vi "TLB Native Dynamic Events ver 0.13c.vi"() -> ()   [LabVIEW 2018]
uses:
  Labview Training Phase 2/Enum Controls/States for Action Engine.ctl
  TLB Type Definitions/State Type Definitions, for 0.26d versions and later.ctl
  TLB Type Definitions/Intruction Type Definitions.ctl
  TLB Type Definitions/Encoder cluster.ctl
  TLB Type Definitions/PING CLUSTER.ctl
  <vilib>/Studica/Studica Toolkit/NavX/NavX.lvlib
  <vilib>/Studica/Studica Toolkit/Background/DIO Channel.ctl
  Underlying VI's/NavX VI/navX type def.ctl
  <vilib>/myRIO/Instrument Drivers/Utilities/Utilities.lvlib
  <vilib>/Studica/Studica Toolkit/Background/I2C Channel.ctl
  TLB Type Definitions/Vision cluster.ctl
  <vilib>/NI_Real-Time Target Support.lvlib
  TLB Type Definitions/Stepper cluster.ctl
  Experimental VI's/Archived VI's/MOTOR CONTROL NO PID Type Def.ctl
  Underlying VI's/I2C Master VI/I2C MASTER Type Def.ctl
  Underlying VI's/I2C Master VI/I2C_MASTER_WRITE_NEW Type Def.ctl
  Underlying VI's/Webcam FGV Low level ver/State control.ctl
  <vilib>/userdefined/High Color/IMAQdx.ctl
  Underlying VI's/I2C Master VI/Arduino_Interfacing.ctl
  <vilib>/Studica/Studica Toolkit/NavX/TypeDefs/Flags/Z900_navX_Flags_CalibrationStatusTypeDef.ctl
  <vilib>/Studica/Studica Toolkit/NavX/TypeDefs/Flags/Z900_navX_Flags_OpStatusTypeDef.ctl
  <vilib>/Utility/RT CPU Load.ctl
panel:
  out "Arduino Data":T1
  out "CPU loads":T2[](array[typedef]) {"ISR (%)" format="%#.2f"; "Idle (%)" format="%#.2f"; "Background (%)" format="%#.2f"; "Normal (%)" format="%#.2f"; "Above Normal (%)" format="%#.2f"; "High (%)" format="%#.2g"; "Timed Structures (%)" format="%#.2g"; "Time Critical (%)" format="%#.2g"; "Total (%)" format="%#.2g"}
  in  "Red LED":bool
  out "Object Center Coordinates":cluster{"x":sgl, "y":sgl}
  out "Object detection cluster":T3
  in  "Mode":enum16{"Ball", "Soap", "Gel", "Pipe", "None"}(ring)
  out "Detect?":bool
  out "Status":T6 {"OP Status" items=["INITIALIZING", "SELFTEST_IN_PROGRESS", "ERROR", "IMU_AUTOCAL_IN_PROGRESS", "NORMAL"]; "Calibration Status" items=["IMU_CAL_STATE_MASK"=3, "IMU_CAL_STATE_INPROGRESS"=0, "IMU_CAL_STATE_ACCUMULATE"=1, "IMU_CAL_STATE_COMPLETE"=2]}
  out "NavX Readings":T7
  out "TASK ENABLE":bool
  out "Rising Edge":bool
  in  "Green LED":bool
  out "Object detected?":bool
  out "I2C Error":errorcluster
  out "Speed & distance":T8
  out "State Logic":T9=enum."Startup"
  out "elements":T10[](array[typedef])
  in  "STOP TASK":bool
  in  "OK Button":bool
  in  "STOP":bool
  out "error out":errorcluster
  out "Action Queue Items":i32
  out "State Logic Queue Items":i32
  out "Action Queues items":string[](array[string])=["Hardware reset", "Software reset", ""]
  out "Action State":string
  # "TLB FRAMEWORK STATUS"
  # "System Health Status Update"
  # "Test Programme written by Calvin Loke    Dated: 28 Aug 2019\nTest Programme revised by Dr Alex See   Dated 30 Aug 2019\n\nProgramme version:   TLB Native Dynamic Events ver 0.04b.vi"
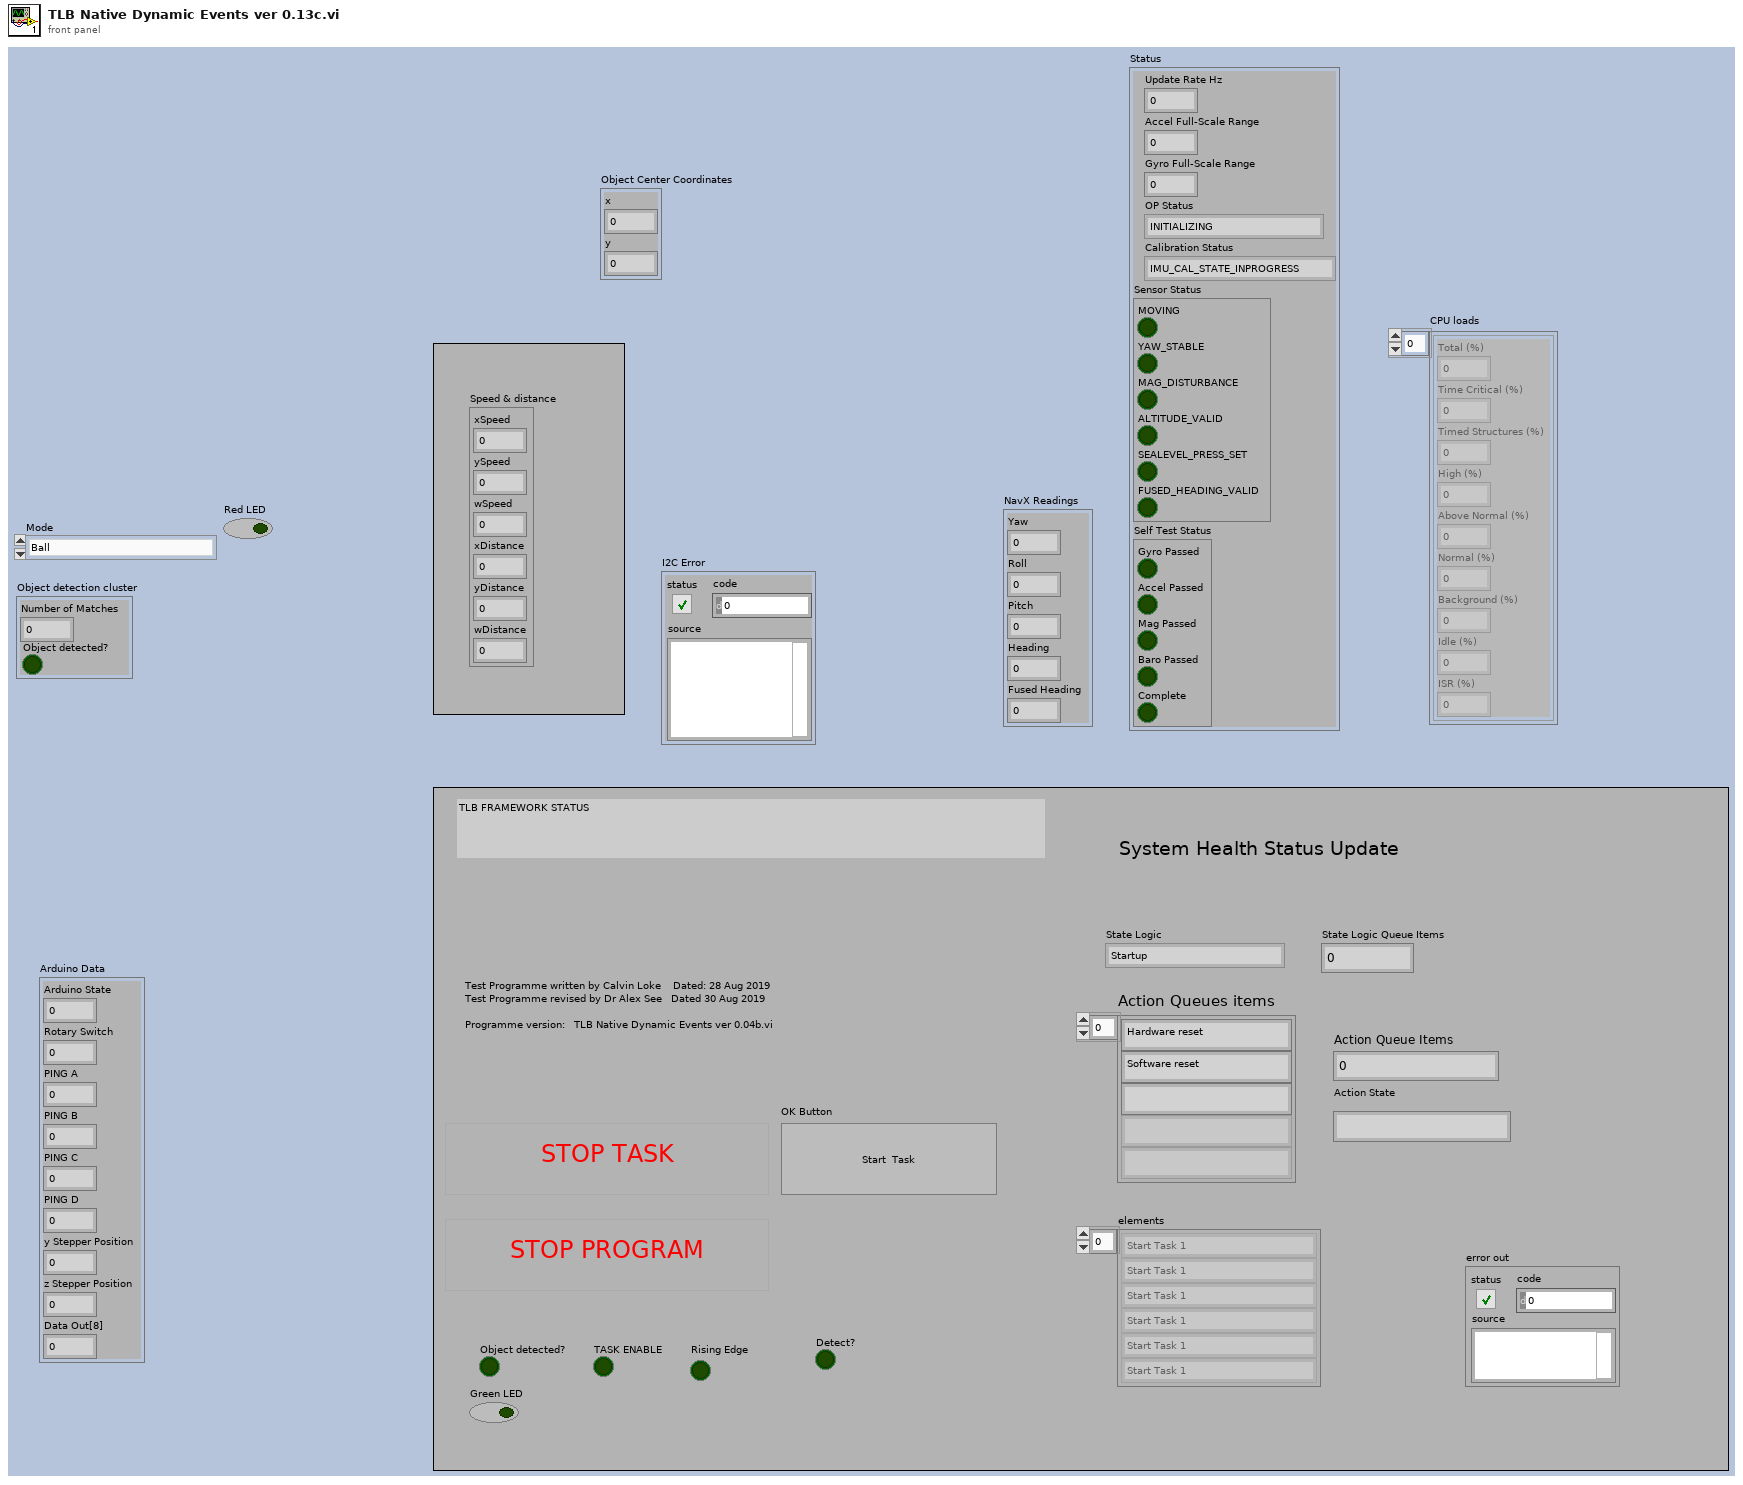
[diagram p1: front panel]
types:
  T1 = cluster{"Arduino State":u8, "Rotary Switch":u8, "PING A":u8, "PING B":u8, "PING C":u8, "PING D":u8, "y Stepper Position":u8, "z Stepper Position":u8, "Data Out[8]":u8}
  T2 = typedef "NI_Real-Time Target Support.lvlib/RT CPU Load.ctl" = cluster{"Total (%)":dbl, "Time Critical (%)":dbl, "Timed Structures (%)":dbl, "High (%)":dbl, "Above Normal (%)":dbl, "Normal (%)":dbl, "Background (%)":dbl, "Idle (%)":dbl, "ISR (%)":dbl}
  T3 = cluster{"Number of Matches":i32, "Object detected?":bool}
  T4 = typedef "NavX.lvlib/Z900_navX_Flags_OpStatusTypeDef.ctl" = u8
  T5 = typedef "NavX.lvlib/Z900_navX_Flags_CalibrationStatusTypeDef.ctl" = u8
  T6 = cluster{"Update Rate Hz":u8, "Accel Full-Scale Range":u8, "Gyro Full-Scale Range":u16, "OP Status":T4, "Calibration Status":T5, "Sensor Status":cluster{"MOVING":bool, "YAW_STABLE":bool, "MAG_DISTURBANCE":bool, "ALTITUDE_VALID":bool, "SEALEVEL_PRESS_SET":bool, "FUSED_HEADING_VALID":bool}, "Self Test Status":cluster{"Gyro Passed":bool, "Accel Passed":bool, "Mag Passed":bool, "Baro Passed":bool, "Complete":bool}}
  T7 = cluster{"Yaw":dbl, "Roll":dbl, "Pitch":dbl, "Heading":dbl, "Fused Heading":dbl}
  T8 = cluster{"xSpeed":dbl, "ySpeed":dbl, "wSpeed":dbl, "xDistance":dbl, "yDistance":dbl, "wDistance":dbl}
  T9 = typedef "State Type Definitions.ctl" = enum16{"None", "Startup", "Move to Angle", "True Stop", "Idle", "Shutdown", "Task 1A", "Task 1B", "Task 2:Raise Arm", "Task 2:Sensor Mode", "Task 2:Reverse Mode", "Task 3", "Task 4_A", "Task 4_B", "Task 4_C", "Task 4_D", "Task 5A", "Task 5B", "Task 5C", "Task 5D", "Task 5E: POSITION ARM", "Task 5F: ARM GRAB HEIGHT", "Task 5G: CLOSE CLAW", "Task 5H: RAISE ARM", "Task 6_A", "Task 6_B", "Task 7", "Task 8A: RAISE ARM", "Task 8B: MOVE TO BOX", "Task 8C: CAM BURST", "Task 8D: PROCESS IMAGE", "Task 8E: ROBOT ADJUST", "Task 8F: CAM BURST 2", "Task 8G: PROCESS IMAGE 2", "Task 8H: ARM ADJUST", "Task 8I: ARM GRAB HEIGHT", "Task 8J: CLOSE CLAW", "Task 8K: RAISE MY SWORD", "Task 9A: Raise Arm", "Task 9B: Rotate to Angle", "Task 9C: Detect Box", "Task 9D: MOVE FORWARD", "Task 9E: MOVE LEFT", "Task 9F: SCAN IMAGE", "Task 9G: PROCESS COLOUR", "Task 9H: MOVE RIGHT", "Task 9I: SCAN IMAGE", "Task 9J: PROCESS COLOUR", "Task 9K: ROTATE 90 CW", "Task 9L: MOVE FORWARD", "Task 9M: MOVE RIGHT", "Task 9N: SCAN IMAGE", "Task 9O: PROCESS COLOUR", "Task 9P: MOVE RIGHT", "Task 9Q: SCAN IMAGE", "Task 9R: PROCESS COLOUR", "Task A1: Raise Arm", "Task A2: Rotate to Angle", "Task A3: Move Forward", "Task A4: Rotate CW 90"}
  T10 = typedef "Intruction Type Definitions.ctl" = enum16{"None", "Start Task 1", "Start Task 2", "Start Task 3", "Start Task 4", "Start Task 5", "Start Task 6", "Start Task 7", "Start Task 8 - BALL", "Start Task 8 - Gel", "Start Task 8 - Pipe", "Start Task 8 - Soap", "Start Task 9", "Start Task A", "Start Task B", "Exit"}
  T11 = typedef "States for Action Engine.ctl" = enum16{"Initialize", "Write", "Read"}
  T12 = typedef "Stepper cluster.ctl" = cluster{"y Stepper Position":u8, "z Stepper Position":u8}
  T13 = typedef "DIO Channel.ctl" = enum16{"Not Connected", "A/DIO1", "A/DIO2", "A/DIO3", "A/DIO4", "A/DIO5", "A/DIO6", "A/DIO7", "A/DIO13", "B/DIO1", "B/DIO2", "B/DIO3", "B/DIO4", "B/DIO5", "B/DIO6", "B/DIO7", "B/DIO13", "C/DIO0", "C/DIO1", "C/DIO2", "C/DIO3", "C/DIO4", "C/DIO5", "C/DIO6", "C/DIO7"}
  T14 = typedef "Vision cluster.ctl" = cluster{"Recognized Object":bool, "Object X coordinate":dbl, "Object Y coordinate":dbl}
  T15 = typedef "PING CLUSTER.ctl" = cluster{"PING_A":u8, "PING_B":u8, "PING_C":u8, "PING_D":u8}
  T16 = typedef "Encoder cluster.ctl" = cluster{"xDistance":dbl, "yDistance":dbl, "wDistance":dbl}
  T17 = typedef "Arduino_Interfacing.ctl" = enum16{"Initialize", "Write to Arduino", "Read From Arduino"}
  T18 = typedef "I2C Channel.ctl" = enum16{"Not Connected", "A", "B"}
  T19 = typedef "navX type def.ctl" = enum16{"Get i2C reference", "Read Values", "Zero Yaw"}
  T20 = typedef "State Type Definitions.ctl" = enum16{"None", "Startup", "Move to Angle", "True Stop", "Idle", "Shutdown", "Task 1", "Task 2:Raise Arm", "Task 2:Sensor Mode", "Task 2:Reverse Mode", "Task 3", "Task 4_A", "Task 4_B", "Task 4_C", "Task 4_D", "Task 5A: ARM CAM HEIGHT", "Task 5B: MOVE TO BOX", "Task 5C: CAM BURST", "Task 5D: PROCESS IMAGE", "Task 5E: POSITION ARM", "Task 5F: ARM GRAB HEIGHT", "Task 5G: CLOSE CLAW", "Task 5H: RAISE ARM", "Task 6_A", "Task 6_B", "Task 7", "Task 8A: RAISE ARM", "Task 8B: MOVE TO BOX", "Task 8C: CAM BURST", "Task 8D: PROCESS IMAGE", "Task 8E: ROBOT ADJUST", "Task 8F: CAM BURST 2", "Task 8G: PROCESS IMAGE 2", "Task 8H: ARM ADJUST", "Task 8I: ARM GRAB HEIGHT", "Task 8J: CLOSE CLAW", "Task 8K: RAISE MY SWORD", "Task 9A: Raise Arm", "Task 9B: Rotate to Angle", "Task 9C: Detect Box", "Task 9D: MOVE FORWARD", "Task 9E: MOVE LEFT", "Task 9F: SCAN IMAGE", "Task 9G: PROCESS COLOUR", "Task 9H: MOVE RIGHT", "Task 9I: SCAN IMAGE", "Task 9J: PROCESS COLOUR", "Task 9K: ROTATE 90 CW", "Task 9L: MOVE FORWARD", "Task 9M: MOVE RIGHT", "Task 9N: SCAN IMAGE", "Task 9O: PROCESS COLOUR", "Task 9P: MOVE RIGHT", "Task 9Q: SCAN IMAGE", "Task 9R: PROCESS COLOUR"}
  T21 = typedef "State Type Definitions.ctl" = enum16{"None", "Startup", "Move to Angle", "True Stop", "Idle", "Shutdown", "Task 1", "Task 2", "Task 3", "Task 4_A", "Task 4_B", "Task 4_C", "Task 5", "Task 6_A", "Task 6_B", "Task 7", "Task 8", "Task 9", "Task A", "Task B"}
  T22 = typedef "MOTOR CONTROL NO PID Type Def.ctl" = enum16{"Init", "Front Back", "Left Right", "Rotate", "Stop", "Latch"}
  T23 = typedef "I2C_MASTER_WRITE_NEW Type Def.ctl" = enum16{"Ultrasonic sensors", "Stepper origin", "zStepper 13.3k", "zStepper 13k", "zStepper 12k", "zStepper 11k", "zStepper 10k", "zStepper 9k", "zStepper 8k", "zStepper 7k", "zStepper 6k", "zStepper 5k", "zStepper 4k", "zStepper 3k", "zStepper 2k", "zStepper 1k", "zStepper 900", "zStepper 800", "zStepper 700", "zStepper 600", "zStepper 500", "zStepper 400", "zStepper 300", "zStepper 200", "zStepper 100", "zStepper 0", "yStepper control", "Open Claw", "Close Claw", "Soft Reset"}
  T24 = typedef "State control.ctl" = enum16{"Initialise", "Start camera", "Continuous Acquisition ", "Stop camera", "Dispose all"}
  T25 = typedef "IMAQdx.ctl" = refnum<k21>
  T26 = cluster{"DIO Channel":T13, "FPGA VI Reference Out":refnum<k20>}
  T27 = cluster{"I2C Ref Out":cluster{"I2C Channel":T18, "FPGA VI Reference Out":refnum<k20>}, "Connected":bool, "Slave Address (7-bit)":u8, "Registry":u8[]}
  T28 = typedef "IMAQ Image.ctl" = refnum<image>
  T29 = typedef "I2C MASTER Type Def.ctl" = enum16{"Last State", "Mode 0", "Mode 1", "Mode 2", "Mode 3", "Mode 4", "Mode 5", "Mode 6", "Mode 7", "Mode 8", "Mode 9", "Mode 10"}
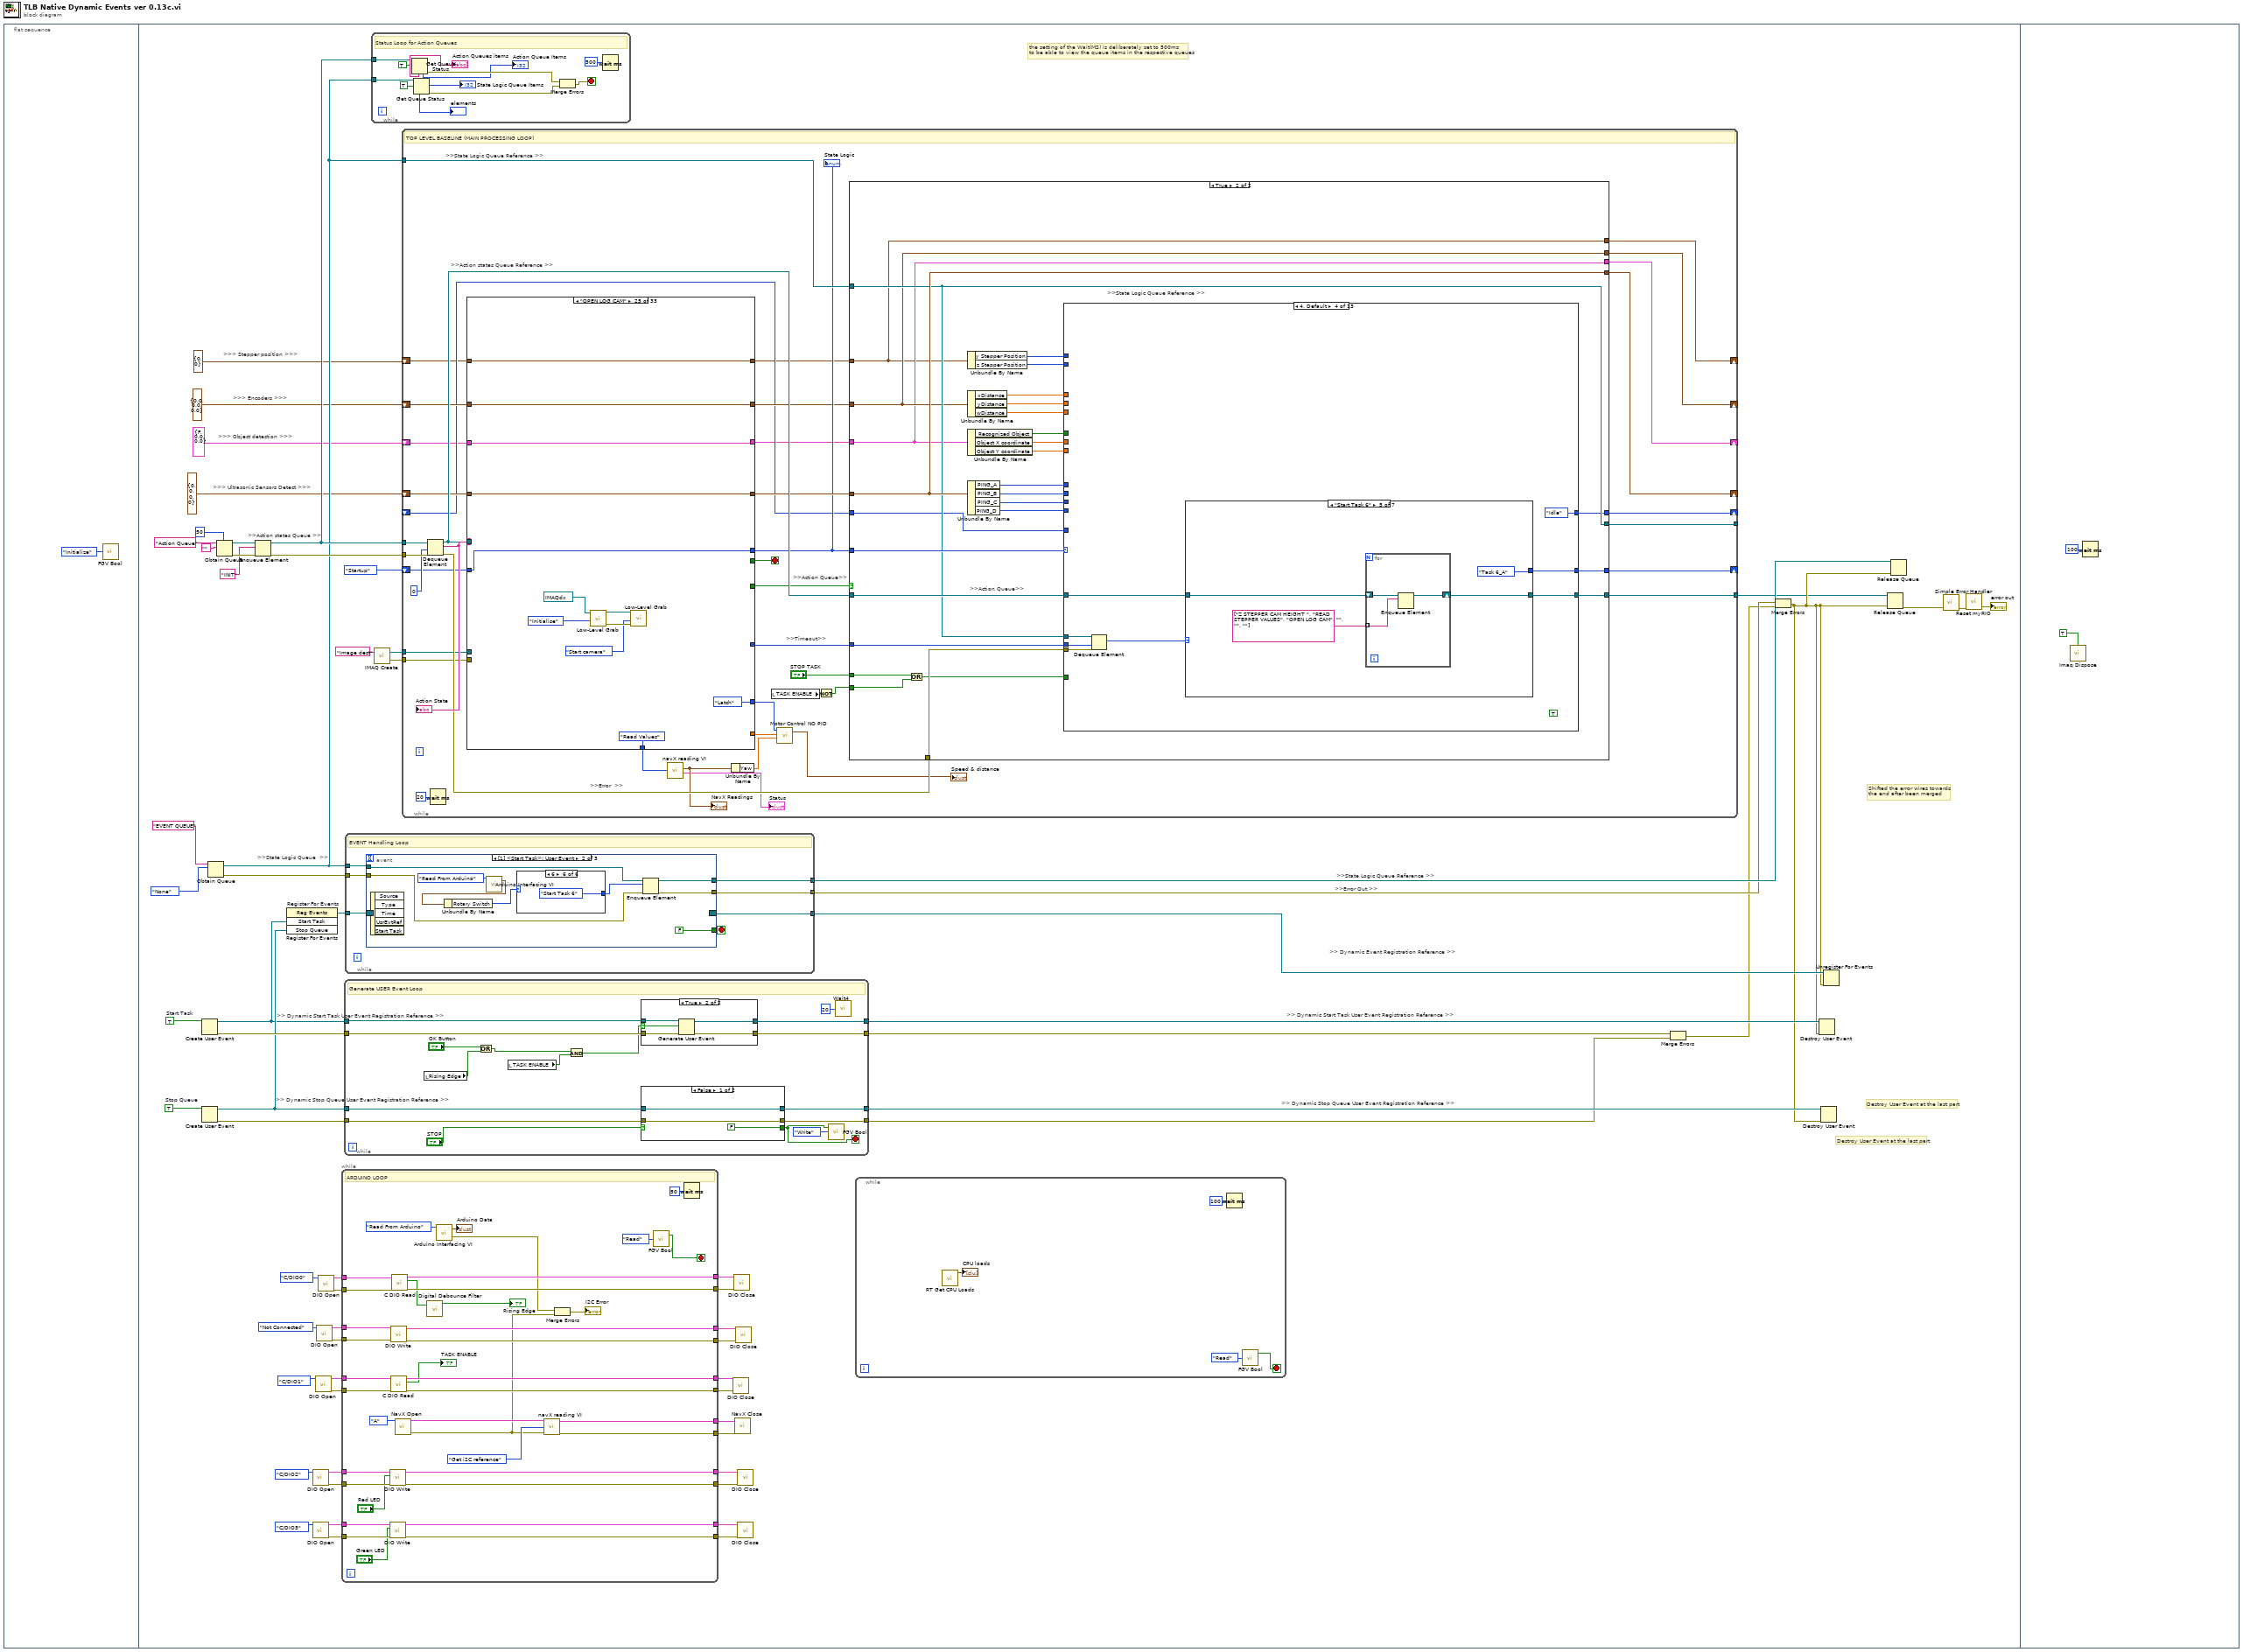
[diagram p0: block diagram]
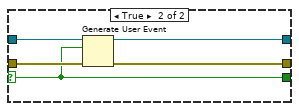
[diagram p2: hidden frame]
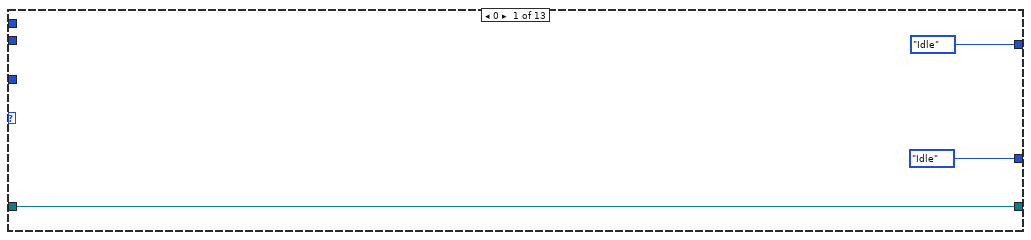
[diagram p5: hidden frame]
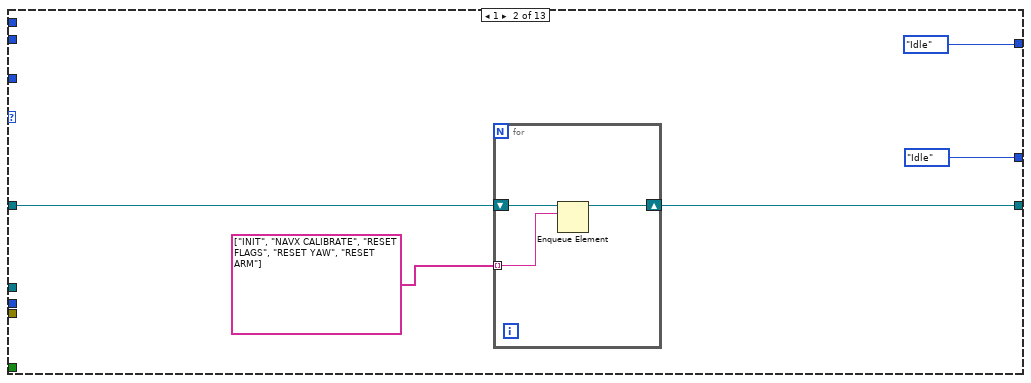
[diagram p6: hidden frame]
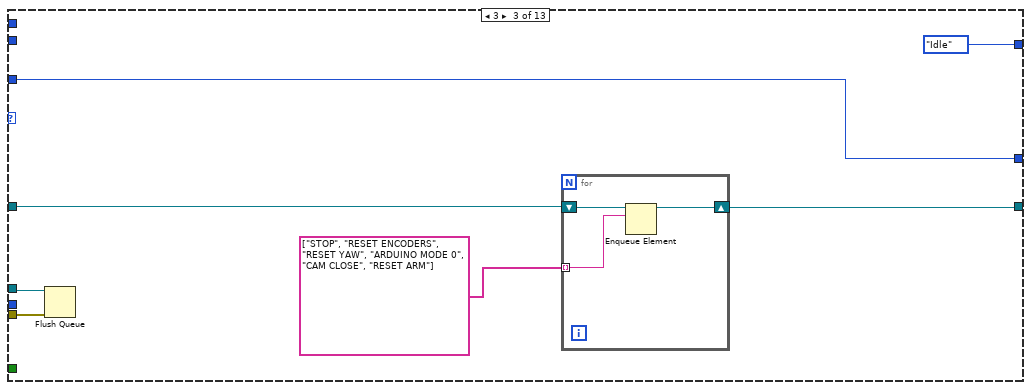
[diagram p7: hidden frame]
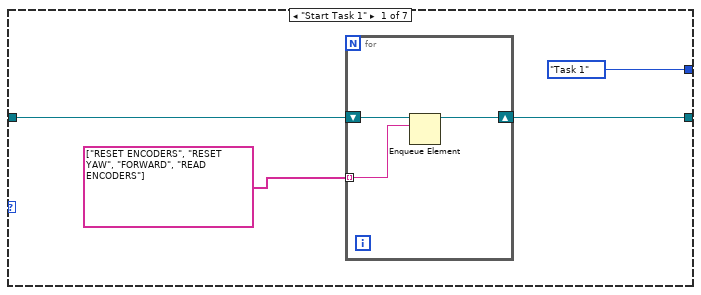
[diagram p8: hidden frame]
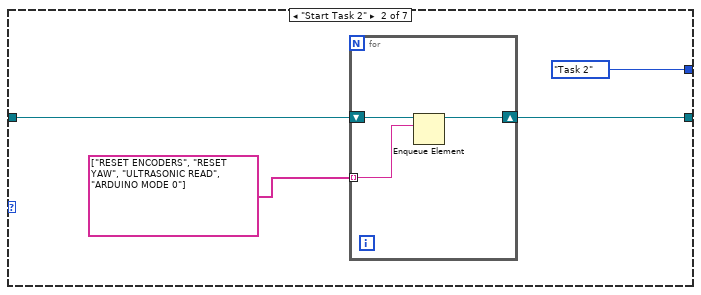
[diagram p9: hidden frame]
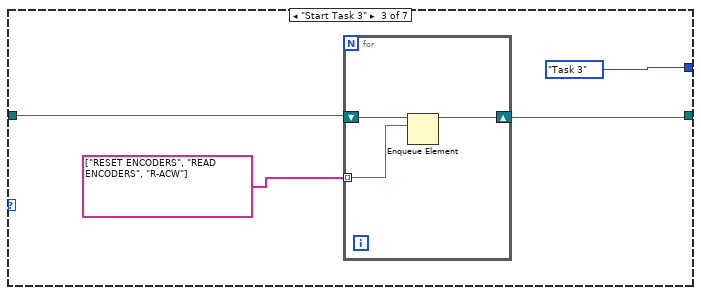
[diagram p10: hidden frame]
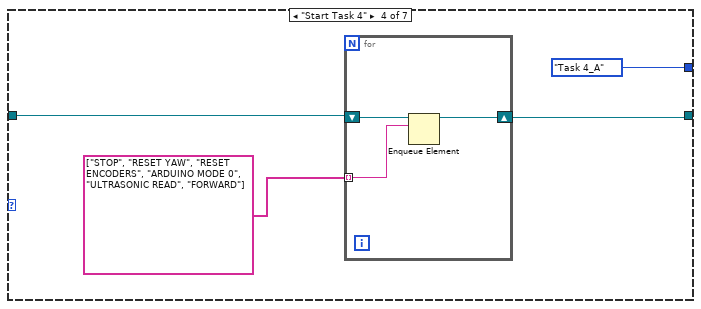
[diagram p11: hidden frame]
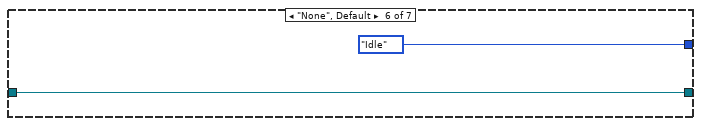
[diagram p12: hidden frame]
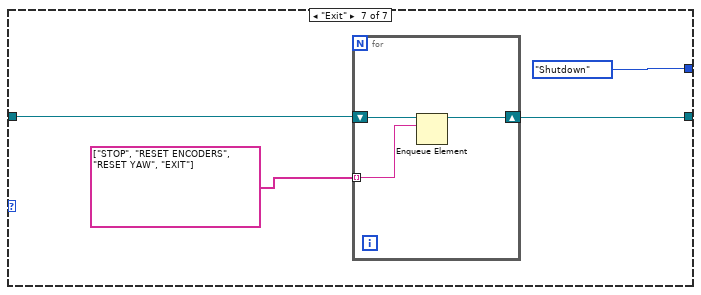
[diagram p13: hidden frame]
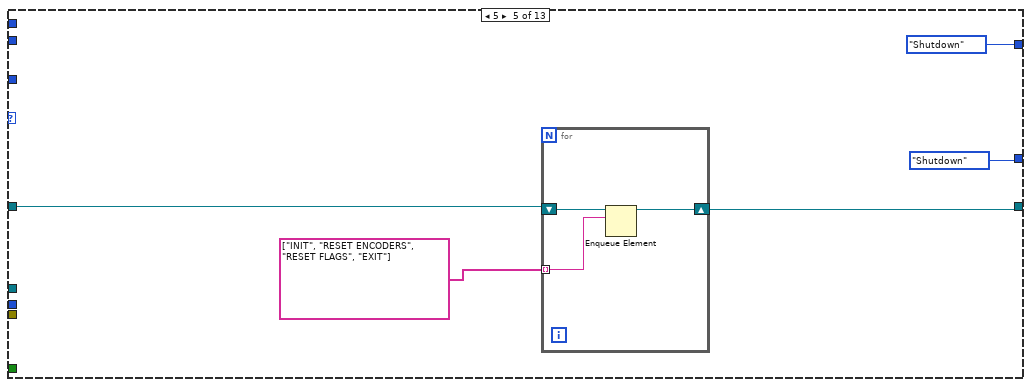
[diagram p14: hidden frame]
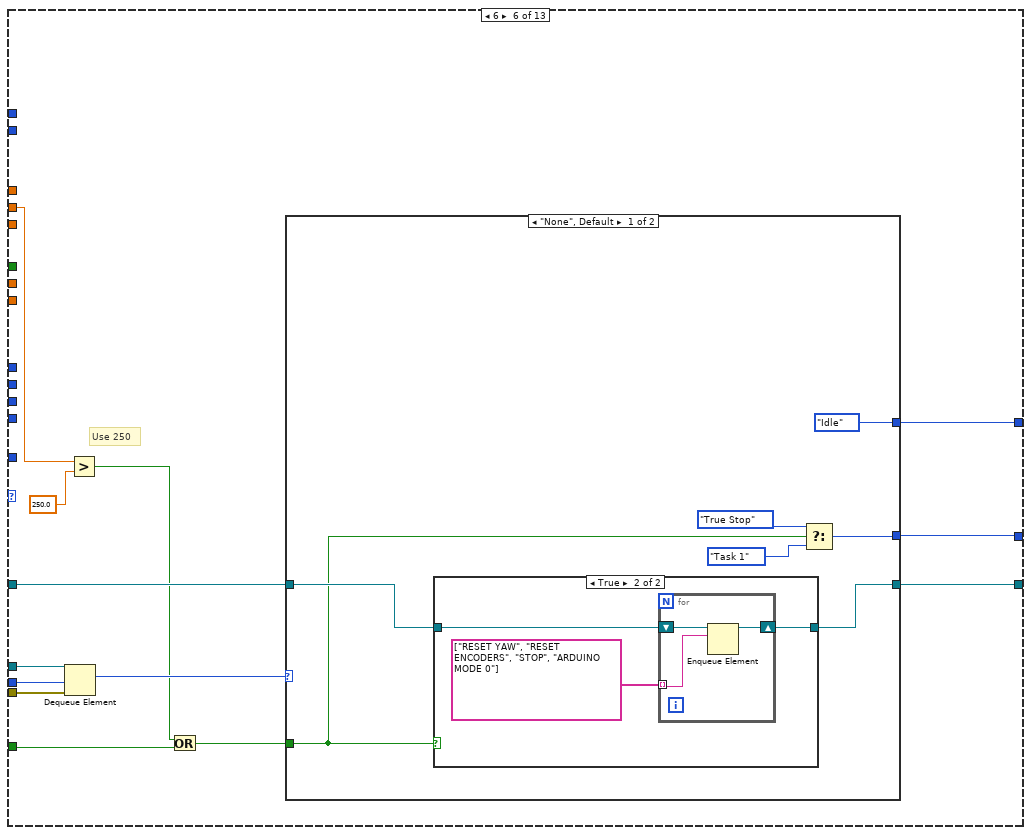
[diagram p15: hidden frame]
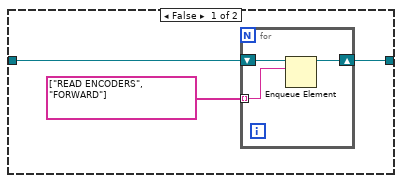
[diagram p16: hidden frame]
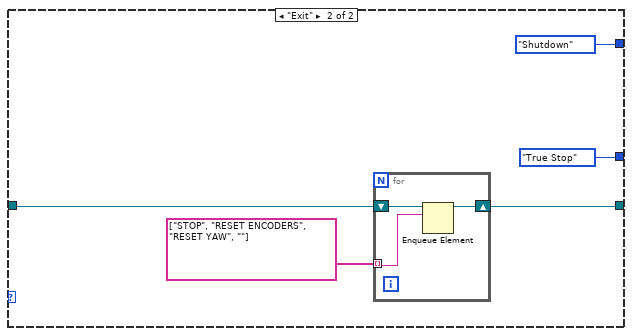
[diagram p17: hidden frame]
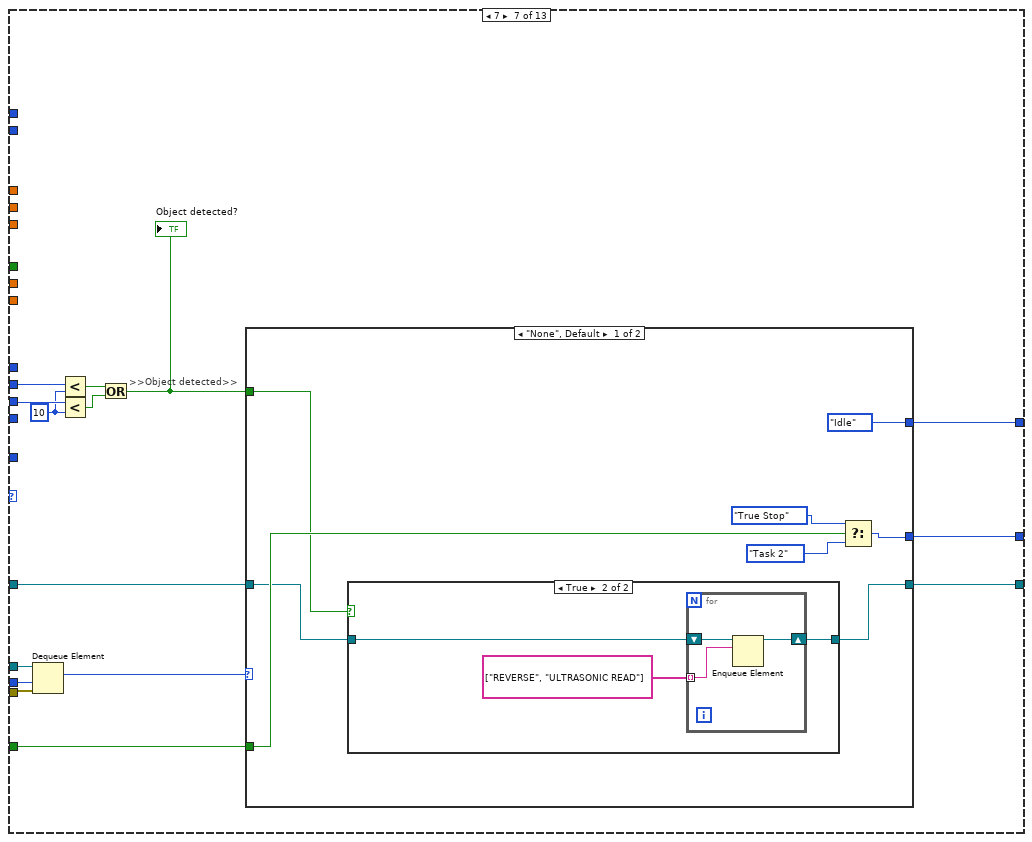
[diagram p18: hidden frame]
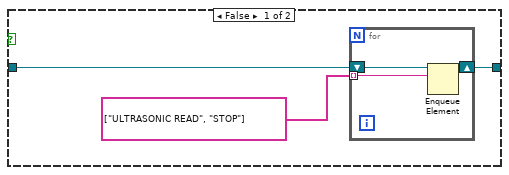
[diagram p19: hidden frame]
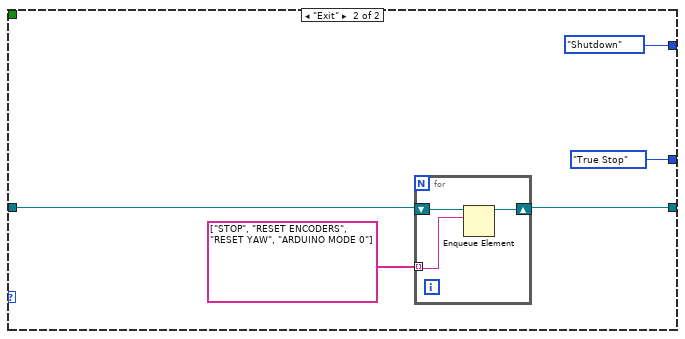
[diagram p20: hidden frame]
diagram:
  n1 = flat-sequence {
    frame #0 {
      n2 = call "FGV Bool.vi"("Init/Read/Write State"=States_for_Action_Engine."Initialize") -> ()  [unwired: 2 in, 2 out]
    }
    frame #1 {
      w68 = TRUE  # Stop Queue
      w67 = TRUE  # Start Task
      # ">>> Stepper position >>>"
      # ">>> Encoders >>>"
      # ">>> Object detection >>>"
      # ">>> Ultrasonic Sensors Detect >>>"
      # "the setting of the Wait(MS) is deliberately set to 500ms\nto be able to view the queue items in the respective queues"
      # ">>Error Out >>"
      # ">> Dynamic Stop Queue User Event Registration Reference >>"
      # ">> Dynamic Start Task User Event Registration Reference >>"
      # ">> Dynamic Stop Queue User Event Registration Reference >>"
      # ">> Dynamic Start Task User Event Registration Reference >>"
      # ">> Dynamic Event Registration Reference >>"
      # ">>Action states Queue >>"
      # ">>State Logic Queue  >>"
      # ">>State Logic Queue Reference >>"
      # "Destroy User Event at the last part"
      # "Destroy User Event at the last part"
      # "Shifted the error wires towards\nthe end after been merged"
      n3 = Create User Event(user event datatype=w67) -> (user event=w59:refnum<user-event>, error out=w64:errorcluster)  [unwired: 1 in]
      n4 = Create User Event(user event datatype=w68) -> (user event=w60:refnum<user-event>, error out=w63:errorcluster)  [unwired: 1 in]
      n5 = Obtain Queue(name (unnamed)="EVENT QUEUE", element data type=Intruction_Type_Definitions."None" ("Enum")) -> (queue out=w45:refnum<queue>, error out=w51:errorcluster)  [unwired: 3 in, 1 out]
      n6 = Obtain Queue(max queue size (-1, unlimited)=50, name (unnamed)="Action Queue", element data type="") -> (queue out=w54:refnum<queue>, error out=w50:errorcluster)  [unwired: 2 in, 1 out]
      n7 = Enqueue Element(queue=w54, element="INIT", error in (no error)=w50) -> (queue out=w46:refnum<queue>, error out=w49:errorcluster)  [unwired: 1 in, 1 out]
      n8 = register-events "Register For Events"(w59, w60) -> (reference out=w58:refnum<event-registration>)  [unwired: 2 in, 1 out]
      n9 = call <vilib>:"DIO Open.vi"("DIO Channel"=DIO_Channel."C/DIO2") -> ("error out"=w10:errorcluster, "DIO Info Out"=w11:T26)  [unwired: 9 in]
      n10 = call <vilib>:"DIO Open.vi"("DIO Channel"=DIO_Channel."C/DIO3") -> ("error out"=w5:errorcluster, "DIO Info Out"=w6:T26)  [unwired: 9 in]
      n11 = call <vilib>:"DIO Open.vi"("DIO Channel"=DIO_Channel."C/DIO1") -> ("error out"=w23:errorcluster, "DIO Info Out"=w24:T26)  [unwired: 9 in]
      n12 = call <vilib>:"DIO Open.vi"("DIO Channel"=DIO_Channel."Not Connected") -> ("error out"=w28:errorcluster, "DIO Info Out"=w30:T26)  [unwired: 9 in]
      n13 = call <vilib>:"DIO Open.vi"("DIO Channel"=DIO_Channel."C/DIO0") -> ("error out"=w33:errorcluster, "DIO Info Out"=w36:T26)  [unwired: 9 in]
      n14 = while {
        tunnel: w36 -> [w107]
        tunnel: [w106] -> w34
        tunnel: w33 -> [w105]
        tunnel: [w104] -> w32
        tunnel: w30 -> [w100]
        tunnel: [w99] -> w29
        tunnel: w28 -> [w98]
        tunnel: [w97] -> w27
        tunnel: [w96] -> w25
        tunnel: w24 -> [w95]
        tunnel: w23 -> [w94]
        tunnel: [w93] -> w22
        tunnel: [w90] -> w21
        tunnel: [w89] -> w20
        tunnel: w11 -> [w85]
        tunnel: w10 -> [w84]
        tunnel: [w83] -> w9
        tunnel: [w82] -> w8
        tunnel: w6 -> [w80]
        tunnel: w5 -> [w79]
        tunnel: [w78] -> w4
        tunnel: [w77] -> w3
        stop <- w109 stop-if-true
        # "ARDUINO LOOP"
        n15 = call <vilib>:"DIO Write.vi"("error in (no error)"=w84, "Input"="Red LED", "DIO Info In"=w85) -> ("error out"=w82:errorcluster, "DIO Info Out"=w83:T26)  [unwired: 7 in]
        n16 = call <vilib>:"DIO Write.vi"("error in (no error)"=w79, "Input"="Green LED", "DIO Info In"=w80) -> ("error out"=w77:errorcluster, "DIO Info Out"=w78:T26)  [unwired: 7 in]
        n17 = call <vilib>:"DIO Write.vi"("error in (no error)"=w98, "DIO Info In"=w100) -> ("error out"=w97:errorcluster, "DIO Info Out"=w99:T26)  [unwired: 8 in]
        n18 = call <vilib>:"C DIO Read.vi"("error in (no error)"=w94, "DIO Info In in"=w95) -> ("error out"=w93:errorcluster, "IN"=→"TASK ENABLE":bool, "DIO Info In out"=w96:T26)  [unwired: 7 in]
        n19 = call <vilib>:"C DIO Read.vi"("error in (no error)"=w105, "DIO Info In in"=w107) -> ("error out"=w104:errorcluster, "IN"=w102:bool, "DIO Info In out"=w106:T26)  [unwired: 7 in]
        n20 = call <vilib>:"NavX Open.vi"("I2C Channel"=I2C_Channel."A") -> ("error out"=w87:errorcluster, "NavX Info"=w91:T27)  [unwired: 9 in]
        n21 = call "Digital Debounce Filter.vi"("Boolean input"=w102) -> ("Rising Edge"=→"Rising Edge":bool)  [unwired: 1 in, 2 out]
        n22 = call "Arduino Interfacing VI.vi"("AE Mode"=Arduino_Interfacing."Read From Arduino") -> ("error out"=w74:errorcluster, "Arduino Data"=→"Arduino Data":T1)  [unwired: 3 in]
        n23 = call "navX reading VI.vi"("NavX Info In"=w91, "Mode"=navX_type_def."Get i2C reference", "error in (no error)"=w87) -> ("NavX Info Out"=w90:T27, "Error Out"=w89:errorcluster)  [unwired: 2 out]
        n24 = Merge Errors(w74, w87) -> (→"I2C Error":errorcluster)
        n25 = call "FGV Bool.vi"("Init/Read/Write State"=States_for_Action_Engine."Read") -> ("Output node"=w109:bool)  [unwired: 2 in, 1 out]
        n26 = Wait (ms)(milliseconds to wait=u32 50) -> ()  [unwired: 1 out]
      }
      n27 = while {
        tunnel: w59 -> [w139]
        tunnel: w60 -> [w138]
        tunnel: [w137] -> w66
        tunnel: [w136] -> w65
        tunnel: w64 -> [w135]
        tunnel: [w134] -> w62
        tunnel: w63 -> [w133]
        tunnel: [w132] -> w61
        stop <- w130 stop-if-true
        # "Generate USER Event Loop"
        n28 = local read "Rising Edge"() -> (w126:bool)
        n29 = Or(x="OK Button", y=w126) -> (x .or. y?=w125:bool)
        n30 = local read "TASK ENABLE"() -> (w124:bool)
        n31 = And(x=w125, y=w124) -> (x .and. y?=w123:bool)
        n32 = case shown="True" w123 {
          selector: w123 -> [_ w150]
          tunnel: w139 -> [w149 w154]
          tunnel: [w149 w153] -> w136
          tunnel: w135 -> [w148 w152]
          tunnel: [w148 w151] -> w134
          frame False {
          }
          frame True {
            n33 = Generate User Event(user event=w154, event data cluster=w150, error in=w152) -> (user event out=w153:refnum<user-event>, error out=w151:errorcluster)  [unwired: 1 in]
          }
        }
        n34 = case shown="False" "STOP" {
          selector: "STOP" -> [_ w143]
          tunnel: w138 -> [w142 w147]
          tunnel: [w142 w146] -> w137
          tunnel: w133 -> [w141 w145]
          tunnel: [w141 w144] -> w132
          tunnel: [FALSE w143] -> w130
          frame False {
          }
          frame True {
            n35 = Generate User Event(user event=w147, event data cluster=w143, error in=w145) -> (user event out=w146:refnum<user-event>, error out=w144:errorcluster)  [unwired: 1 in]
          }
        }
        n36 = call "FGV Bool.vi"("Init/Read/Write State"=States_for_Action_Engine."Write", "Input Node"=w130) -> ()  [unwired: 1 in, 2 out]
        n37 = call "Wait4"("Count(uSec)"=u32 20) -> ()  [unwired: 1 out]
      }
      n38 = while {
        tunnel: w58 -> [w947]
        tunnel: [w946] -> w57
        tunnel: w45 -> [w944]
        tunnel: [w943] -> w56
        tunnel: w51 -> [w942]
        tunnel: [w941] -> w48
        stop <- w945 stop-if-true
        # "EVENT Handling Loop"
        n39 = event shown="[1] <Start Task>: User Event" {
          selector: w947 -> [_ _ _]
          dyn-events: [_ _ _] -> w946
          timeout: _ -> [_ _ _]
          tunnel: [FALSE FALSE w974] -> w945
          tunnel: w944 -> [w952 w961 w972]
          tunnel: [w951 w960 w973] -> w943
          tunnel: w942 -> [w950 w959 w971]
          tunnel: [w949 w958 w970] -> w941
          event Timeout {
            n40 = event-data() -> ()  [unwired: 1 in, 3 out]
            n41 = Enqueue Element(queue=w952, element=Intruction_Type_Definitions."None" ("Enum"), error in (no error)=w950) -> (queue out=w951:refnum<queue>, error out=w949:errorcluster)  [unwired: 1 in, 1 out]
          }
          event User Event {
            n42 = event-data() -> ()  [unwired: 1 in, 5 out]
            n43 = call "Arduino Interfacing VI.vi"("AE Mode"=Arduino_Interfacing."Read From Arduino") -> ("Arduino Data"=w955:T1)  [unwired: 3 in, 1 out]
            n44 = Unbundle By Name(w955) -> ("Rotary Switch"=w954:u8)
            n45 = case shown="6" w954 {
              tunnel: [Intruction_Type_Definitions."None" ("Enum") Intruction_Type_Definitions."Start Task 1" ("Enum") Intruction_Type_Definitions."Start Task 2" ("Enum") Intruction_Type_Definitions."Start Task 3" ("Enum") Intruction_Type_Definitions."Start Task 4" ("Enum") Intruction_Type_Definitions."Start Task 6" ("Enum")] -> w957
              frame 0, Default {
              }
              frame 1 {
              }
              frame 2 {
              }
              frame 3 {
              }
              frame 4 {
              }
              frame 6 {
              }
            }
            n46 = Enqueue Element(queue=w961, element=w957, error in (no error)=w959) -> (queue out=w960:refnum<queue>, error out=w958:errorcluster)  [unwired: 1 in, 1 out]
          }
          event User Event {
            n47 = event-data() -> ("Stop Queue"=w974:bool)  [unwired: 1 in, 4 out]
            n48 = Enqueue Element At Opposite End(queue=w972, element=Intruction_Type_Definitions."Exit" ("Enum"), error in (no error)=w971) -> (queue out=w973:refnum<queue>, error out=w970:errorcluster)  [unwired: 1 in, 1 out]
          }
        }
      }
      n49 = while {
        tunnel: w46 -> [w120]
        tunnel: w45 -> [w117]
        stop <- w114 stop-if-true
        # "Status Loop for Action Queues"
        n50 = Get Queue Status(queue=w120, return elements? (F)=TRUE) -> (error out=w116:errorcluster, # elements in queue=→"Action Queue Items":i32, elements=→"Action Queues items":string[])  [unwired: 1 in, 5 out]
        n51 = Get Queue Status(queue=w117, return elements? (F)=TRUE) -> (# pending remove=→"State Logic Queue Items":i32, error out=w115:errorcluster, elements=→"elements":T10[])  [unwired: 1 in, 5 out]
        n52 = Merge Errors(w116, w115) -> (w114:errorcluster)
        n53 = Wait (ms)(milliseconds to wait=u32 500) -> ()  [unwired: 1 out]
      }
      n54 = call "IMAQ Create"("Image Name"="Image dest") -> ("New Image"=w15:T28, "error out"=w14:errorcluster)  [unwired: 4 in]
      n55 = while {
        tunnel: w45 -> [w184]
        tunnel: w46 -> [w196]
        tunnel: w49 -> [w194]
        tunnel: [w193] -> _
        tunnel: [w192] -> w39
        shift-right: [w185] -> _
        shift-left: T15 {"PING_A"=0, "PING_B"=0, "PING_C"=0, "PING_D"=0} -> [w187]
        shift-right: [w178] -> _
        shift-left: State_Type_Definitions."Startup" ("Enum") -> [w181]
        shift-right: [w174] -> _
        shift-left: T16 {"xDistance"=0.0, "yDistance"=0.0, "wDistance"=0.0} -> [w176]
        shift-right: [w168] -> _
        shift-left: _ -> [w167]
        tunnel: w15 -> [w162]
        tunnel: w14 -> [w161]
        shift-right: [w158] -> _
        shift-left: T14 {"Recognized Object"=FALSE, "Object X coordinate"=0.0, "Object Y coordinate"=0.0} -> [w160]
        shift-right: [w155] -> _
        shift-left: T12 {"y Stepper Position"=0, "z Stepper Position"=0} -> [w157]
        stop <- w183 stop-if-true
        # ">>Error  >>"
        # ">>Action Queue>>"
        # ">>Timeout>>"
        # ">>Action states Queue Reference >>"
        # ">>State Logic Queue Reference >>"
        # "TOP LEVEL BASELINE (MAIN PROCESSING LOOP)"
        n56 = Dequeue Element(queue=w196, timeout in ms (-1)=0, error in (no error)=w194) -> (queue out=w188:refnum<queue>, element=w195:string, error out=w189:errorcluster)  [unwired: 1 out]
        "Action State" <- w195
        n57 = Wait (ms)(milliseconds to wait=u32 20) -> ()  [unwired: 1 out]
        n58 = case shown="\"OPEN LOG CAM\"" w195 {
          tunnel: [_ _ _ _ _ _ _ _ _ _ _ _ _ _ _ _ 0 w799 _ _ _ _ _ _ _ _ _ _ _ _ _ _ _] -> w191
          tunnel: w188 -> [_ _ _ _ _ _ _ _ _ _ _ _ _ _ _ _ _ _ _ _ _ _ _ _ _ _ _ _ _ _ _ _ _]
          tunnel: w187 -> [w665 w671 w679 w686 w693 w699 w707 w715 w722 w726 w739 w752 w757 w772 w777 w782 w791 w800 w806 w812 w831 w840 w845 w851 w863 w875 w892 w903 w907 w914 w921 w928 w938]
          tunnel: [w665 w671 w679 w686 w693 w699 w707 w715 w722 w726 w739 w753 w757 w773 w777 w782 w791 w800 w806 w812 w830 w840 w845 w851 w863 w875 w892 w903 w907 w914 w921 w928 w938] -> w186
          tunnel: [TRUE TRUE _ _ _ _ _ _ _ _ _ _ _ _ _ _ _ _ _ _ _ _ _ _ _ _ _ _ _ _ _ _ _] -> w183
          tunnel: w181 -> [w663 w669 w678 w685 w692 w698 w706 w714 w721 w725 w738 w751 w756 w771 w776 w781 w788 w797 w805 w811 w829 w839 w844 w850 w857 w869 w891 w898 w906 w913 w920 w927 w937]
          tunnel: [_ _ _ _ _ _ _ _ _ _ _ _ _ _ _ _ _ TRUE _ _ _ _ _ _ _ _ _ _ _ _ _ _ _] -> w180
          tunnel: [w663 w669 w678 w685 w692 w698 w706 w714 w721 w725 w738 w751 w756 w771 w776 w781 w788 w797 w805 w811 w829 w839 w844 w850 w857 w869 w891 w898 w906 w913 w920 w927 w937] -> w179
          tunnel: w176 -> [w662 w668 w677 w684 w691 w697 w705 w713 w720 w727 w737 w750 w758 w770 w778 w783 w787 w796 w807 w813 w819 w838 w847 w852 w864 w876 w893 w904 w909 w916 w923 w930 w940]
          tunnel: [w662 w668 w677 w684 w691 w697 w705 w713 w720 w727 w736 w750 w758 w769 w778 w783 w787 w796 w807 w813 w818 w838 w847 w852 w864 w876 w893 w904 w909 w916 w923 w930 w940] -> w175
          tunnel: [_ _ 0.4 ("Speed") -0.3 ("Speed") 0.19999999999999998 ("Speed") -0.2 ("Speed") _ 0.3 ("Speed") -0.5 ("Speed") _ _ _ _ 0.0 ("Speed") _ _ _ _ _ _ _ _ _ _ _ _ _ _ _ _ _ _ _] -> w173
          tunnel: [_ _ MOTOR_CONTROL_NO_PID_Type_Def."Front Back" ("Direction") _ MOTOR_CONTROL_NO_PID_Type_Def."Rotate" ("Direction") _ MOTOR_CONTROL_NO_PID_Type_Def."Stop" ("Direction") MOTOR_CONTROL_NO_PID_Type_Def."Left Right" ("Direction") MOTOR_CONTROL_NO_PID_Type_Def."Front Back" ("Direction") _ MOTOR_CONTROL_NO_PID_Type_Def."Latch" ("Direction") MOTOR_CONTROL_NO_PID_Type_Def."Latch" ("Direction") _ _ _ _ _ MOTOR_CONTROL_NO_PID_Type_Def."Latch" ("Direction") _ MOTOR_CONTROL_NO_PID_Type_Def."Init" ("Direction") _ MOTOR_CONTROL_NO_PID_Type_Def."Init" ("Direction") _ _ MOTOR_CONTROL_NO_PID_Type_Def."Latch" ("Direction") MOTOR_CONTROL_NO_PID_Type_Def."Latch" ("Direction") _ MOTOR_CONTROL_NO_PID_Type_Def."Latch" ("Direction") _ _ _ _ _] -> w171
          tunnel: [_ _ navX_type_def."Read Values" ("Mode") navX_type_def."Read Values" ("Mode") _ _ navX_type_def."Read Values" ("Mode") navX_type_def."Read Values" ("Mode") _ _ navX_type_def."Read Values" ("Mode") navX_type_def."Read Values" ("Mode") _ navX_type_def."Zero Yaw" ("Mode") _ _ navX_type_def."Zero Yaw" ("Mode") navX_type_def."Read Values" ("Mode") _ _ _ navX_type_def."Zero Yaw" ("Mode") _ _ navX_type_def."Read Values" ("Mode") navX_type_def."Read Values" ("Mode") _ navX_type_def."Read Values" ("Mode") _ _ _ _ _] -> w165
          tunnel: w162 -> [_ _ _ _ _ _ _ _ _ _ _ _ _ _ _ _ _ _ _ _ _ _ _ _ _ _ w886 _ _ _ _ _ _]
          tunnel: w161 -> [_ _ _ _ _ _ _ _ _ _ _ _ _ _ _ _ _ _ _ _ _ _ _ _ _ _ w885 _ _ _ _ _ _]
          tunnel: w160 -> [w661 w667 w673 w681 w688 w695 w701 w709 w717 w724 w729 w747 w755 w764 w775 w780 w785 w793 w804 w809 w824 w834 w846 w849 w854 w866 w884 w895 w908 w915 w922 w929 w939]
          tunnel: [w661 w667 w673 w681 w688 w695 w701 w709 w717 w724 w729 w747 w755 w764 w775 w780 w785 w793 w804 w809 w823 w834 w846 w849 w854 w866 w878 w895 w908 w915 w922 w929 w939] -> w159
          tunnel: w157 -> [w660 w666 w672 w680 w687 w694 w700 w708 w716 w723 w728 w746 w754 w763 w774 w779 w784 w792 w803 w808 w814 w833 w843 w848 w853 w865 w877 w894 w905 w912 w919 w926 w936]
          tunnel: [w660 w666 w672 w680 w687 w694 w700 w708 w716 w723 w728 w746 w754 w762 w774 w779 w784 w792 w803 w808 w814 w833 w843 w848 w853 w865 w877 w894 w905 w912 w919 w926 w935] -> w156
          frame "Exit" {
          }
          frame "----Movement States----" {
          }
          frame "FORWARD" {
          }
          frame "LEFT" {
            (unwired) I2C_MASTER_Type_Def."Last State" ("Arduino Mode")
          }
          frame "R-ACW" {
            (unwired) I2C_MASTER_Type_Def."Last State" ("Arduino Mode")
          }
          frame "R-CW" {
            (unwired) I2C_MASTER_Type_Def."Last State" ("Arduino Mode")
          }
          frame "STOP" {
            (unwired) I2C_MASTER_Type_Def."Last State" ("Arduino Mode")
            n59 = Wait (ms)(milliseconds to wait=u32 200) -> ()  [unwired: 1 out]
          }
          frame "RIGHT" {
            (unwired) I2C_MASTER_Type_Def."Last State" ("Arduino Mode")
          }
          frame "REVERSE" {
            (unwired) I2C_MASTER_Type_Def."Last State" ("Arduino Mode")
          }
          frame "----SENSOR READING---- " {
            (unwired) I2C_MASTER_Type_Def."Last State" ("Arduino Mode")
          }
          frame "READ ENCODERS" {
            (unwired) I2C_MASTER_Type_Def."Last State" ("Arduino Mode")
            # ">>> Current encoder distance >>>"
            # ">>> Ultrasonic Sensors Detect >>>"
            n60 = local read "Speed & distance"() -> (w735:T8)
            n61 = Unbundle By Name(w735) -> ("xDistance"=w734:dbl, "yDistance"=w733:dbl, "wDistance"=w732:dbl)
            n62 = Bundle By Name(cluster=w737, "xDistance"=w734, "yDistance"=w733, "wDistance"=w732) -> (w736:T16)
          }
          frame "ULTRASONIC READ" {
            # "Object detection"
            n63 = call "Arduino Interfacing VI.vi"("AE Mode"=Arduino_Interfacing."Read From Arduino") -> ("Arduino Data"=w744:T1)  [unwired: 3 in, 1 out]
            n64 = Unbundle By Name(w744) -> ("PING A"=w743:u8, "PING B"=w742:u8, "PING C"=w741:u8, "PING D"=w740:u8)
            n65 = Bundle By Name(cluster=w752, "PING_A"=w743, "PING_B"=w742, "PING_C"=w741, "PING_D"=w740) -> (w753:T15)
          }
          frame "----SYSTEM MODES----" {
            (unwired) I2C_MASTER_Type_Def."Last State" ("Arduino Mode")
          }
          frame "INIT" {
            (unwired) I2C_MASTER_Type_Def."Last State" ("Arduino Mode")
            w766 = u8 0
            w768 = 0.0
            # ">>State Logic  >>"
            n66 = Bundle By Name(cluster=w772, "PING_A"=w766, "PING_B"=w766, "PING_C"=w766, "PING_D"=w766) -> (w773:T15)
            n67 = Bundle By Name(cluster=w763, "y Stepper Position"=u8 0, "z Stepper Position"=u8 0) -> (w762:T12)
            n68 = Bundle By Name(cluster=w770, "xDistance"=w768, "yDistance"=w768, "wDistance"=w768) -> (w769:T16)
            n69 = call "Arduino Interfacing VI.vi"("AE Mode"=Arduino_Interfacing."Initialize") -> ()  [unwired: 3 in, 2 out]
          }
          frame "ARDUINO MODE 0" {
            (unwired) I2C_MASTER_WRITE_NEW_Type_Def."Ultrasonic sensors" ("Arduino mode")
          }
          frame "ARDUINO MODE 1" {
            (unwired) I2C_MASTER_Type_Def."Mode 1" ("Arduino Mode")
          }
          frame "NAVX CALIBRATE" {
            (unwired) I2C_MASTER_Type_Def."Last State" ("Arduino Mode")
            # "Adds a 15 second delay to the startup process \nfor the NavX to calibrate"
            n70 = Wait (ms)(milliseconds to wait=u32 5000) -> ()  [unwired: 1 out]
          }
          frame "NO ACTION", Default {
            (unwired) u8 0 ("y Stepper value")
            (unwired) TRUE ("Latch")
            n71 = case shown="4" w797 {
              tunnel: [0 100] -> w799
              frame 1, Default {
              }
              frame 4 {
              }
            }
          }
          frame "----RESET CASES----" {
            (unwired) I2C_MASTER_Type_Def."Last State" ("Arduino Mode")
          }
          frame "RESET ENCODERS" {
            (unwired) I2C_MASTER_Type_Def."Last State" ("Arduino Mode")
          }
          frame "RESET FLAGS" {
            (unwired) I2C_MASTER_Type_Def."Last State" ("Arduino Mode")
            # "Resets any software variables\nand/or non-critical states"
            n72 = Wait (ms)(milliseconds to wait=u32 20) -> ()  [unwired: 1 out]
            n73 = Bundle By Name(cluster=w819, "xDistance"=0.0, "yDistance"=0.0, "wDistance"=0.0) -> (w818:T16)
            n74 = Bundle By Name(cluster=w824, "Recognized Object"=FALSE, "Object X coordinate"=0.0, "Object Y coordinate"=0.0) -> (w823:T14)
            n75 = Bundle By Name(cluster=w831, "PING_A"=u8 0, "PING_B"=u8 0, "PING_C"=u8 0, "PING_D"=u8 0) -> (w830:T15)
          }
          frame "RESET YAW" {
            (unwired) I2C_MASTER_Type_Def."Last State" ("Arduino Mode")
            n76 = Wait (ms)(milliseconds to wait=u32 100) -> ()  [unwired: 1 out]
          }
          frame "RESET ARM" {
            n77 = call "Arduino Interfacing VI.vi"("Data to Write"=I2C_MASTER_WRITE_NEW_Type_Def."Soft Reset", "AE Mode"=Arduino_Interfacing."Write to Arduino") -> ()  [unwired: 2 in, 2 out]
          }
          frame "--------CAM STATES-------" {
          }
          frame "OPEN LOG CAM" {
            n78 = call "Low-Level Grab.vi"("States"=State_control."Initialise", "Session In"=T25 "cam0") -> ("error out"=w859:errorcluster, "Session Out"=w860:T25)  [unwired: 7 in, 1 out]
            n79 = call "Low-Level Grab.vi"("error in (no error)"=w859, "States"=State_control."Start camera", "Session In"=w860) -> ()  [unwired: 6 in, 3 out]
          }
          frame "OPEN LIFE CAM" {
            n80 = call "Low-Level Grab.vi"("States"=State_control."Initialise", "Session In"=T25 "cam1") -> ("error out"=w871:errorcluster, "Session Out"=w872:T25)  [unwired: 7 in, 1 out]
            n81 = call "Low-Level Grab.vi"("error in (no error)"=w871, "States"=State_control."Start camera", "Session In"=w872) -> ()  [unwired: 6 in, 3 out]
          }
          frame "CAM ACQ" {
            n82 = call "Low-Level Grab.vi"("error in (no error)"=w885, "States"=State_control."Continuous Acquisition ") -> ("error out"=w888:errorcluster, "Image Out"=w889:T28)  [unwired: 7 in, 1 out]
            n83 = call "Object Detection SubVI.vi"("Error In"=w888, "Mode"="Mode", "Image Dest"=w886, "Image in"=w889) -> ("Object Center Coordinates"=w883:cluster{"x":sgl, "y":sgl}, "Object detection cluster"=w880:T3)  [unwired: 2 out]
            "Object detection cluster" <- w880
            "Object Center Coordinates" <- w883
            n84 = Unbundle By Name(w880) -> ("Object detected?"=w879:bool)
            n85 = Unbundle By Name(w883) -> ("x"=w882:sgl, "y"=w881:sgl)
            n86 = Bundle By Name(cluster=w884, "Recognized Object"=w879, "Object X coordinate"=w882, "Object Y coordinate"=w881) -> (w878:T14)
          }
          frame "CAM CLOSE" {
            n87 = call "Low-Level Grab.vi"("States"=State_control."Stop camera") -> ("error out"=w900:errorcluster, "Session Out"=w901:T25)  [unwired: 8 in, 1 out]
            n88 = call "Low-Level Grab.vi"("error in (no error)"=w900, "States"=State_control."Dispose all", "Session In"=w901) -> ()  [unwired: 6 in, 3 out]
          }
          frame "-----ARM ACTIONS-----" {
          }
          frame "CLOSE CLAW" {
            n89 = call "Arduino Interfacing VI.vi"("Data to Write"=I2C_MASTER_WRITE_NEW_Type_Def."Close Claw", "AE Mode"=Arduino_Interfacing."Write to Arduino") -> ()  [unwired: 2 in, 2 out]
          }
          frame "OPEN CLAW" {
            n90 = call "Arduino Interfacing VI.vi"("Data to Write"=I2C_MASTER_WRITE_NEW_Type_Def."Open Claw", "AE Mode"=Arduino_Interfacing."Write to Arduino") -> ()  [unwired: 2 in, 2 out]
          }
          frame "Z STEPPER CAM HEIGHT " {
            n91 = call "Arduino Interfacing VI.vi"("Data to Write"=I2C_MASTER_WRITE_NEW_Type_Def."zStepper 10k", "AE Mode"=Arduino_Interfacing."Write to Arduino") -> ()  [unwired: 2 in, 2 out]
          }
          frame "READ STEPPER VALUES" {
            n92 = call "Arduino Interfacing VI.vi"("AE Mode"=Arduino_Interfacing."Read From Arduino") -> ("Arduino Data"=w933:T1)  [unwired: 3 in, 1 out]
            n93 = Unbundle By Name(w933) -> ("y Stepper Position"=w932:u8, "z Stepper Position"=w931:u8)
            n94 = Bundle By Name(cluster=w936, "y Stepper Position"=w932, "z Stepper Position"=w931) -> (w935:T12)
          }
        }
        "State Logic" <- w179
        n95 = call "navX reading VI.vi"("Mode"=w165) -> ("NavX Readings"=w166:T7, "Status"=→"Status":T6)  [unwired: 2 in, 2 out]
        "NavX Readings" <- w166
        n96 = Unbundle By Name(w166) -> ("Yaw"=w164:dbl)
        n97 = local read "TASK ENABLE"() -> (w170:bool)
        n98 = call "Motor Control NO PID.vi"("Yaw"=w164, "Speed"=w173, "Direction"=w171) -> ("Speed & distance"=→"Speed & distance":T8)  [unwired: 1 in, 1 out]
        n99 = Not(x=w170) -> (.not. x?=w169:bool)
        n100 = case shown="True" w180 {
          tunnel: w184 -> [w204 w227]
          tunnel: w188 -> [w200 w229]
          tunnel: [w204 w227] -> w193
          tunnel: [w200 w230] -> w192
          tunnel: w189 -> [_ w225]
          tunnel: w191 -> [_ w226]
          tunnel: w186 -> [w203 w232]
          tunnel: [w203 w232] -> w185
          tunnel: "STOP TASK" -> [_ w215]
          tunnel: w179 -> [w202 w231]
          tunnel: [w202 w228] -> w178
          tunnel: w175 -> [w201 w221]
          tunnel: [w201 w221] -> w174
          tunnel: w169 -> [_ w216]
          tunnel: [w199 w213] -> w168
          tunnel: w167 -> [w199 w212]
          tunnel: w159 -> [w198 w209]
          tunnel: [w198 w209] -> w158
          tunnel: w156 -> [w197 w205]
          tunnel: [w197 w205] -> w155
          frame False {
          }
          frame True {
            # ">>Action Queue>>"
            # ">>State Logic Queue Reference >>"
            n101 = Or(x=w215, y=w216) -> (x .or. y?=w214:bool)
            n102 = Unbundle By Name(w205) -> ("y Stepper Position"=w207:u8, "z Stepper Position"=w206:u8)
            n103 = Unbundle By Name(w221) -> ("xDistance"=w218:dbl, "yDistance"=w219:dbl, "wDistance"=w220:dbl)
            n104 = Unbundle By Name(w209) -> ("Recognized Object"=w208:bool, "Object X coordinate"=w211:dbl, "Object Y coordinate"=w210:dbl)
            n105 = Unbundle By Name(w232) -> ("PING_A"=w224:u8, "PING_B"=w223:u8, "PING_C"=w222:u8, "PING_D"=w217:u8)
            n106 = case shown="4, Default" w231 {
              tunnel: [w234 w237 w248 w255 w307 w319 w355 w401 w445 w502 w539 w591 w632] -> w230
              tunnel: w229 -> [w234 w240 w249 w258 w309 w320 w356 w402 w451 w495 w543 w586 w623]
              tunnel: [State_Type_Definitions."Idle" ("Enum") State_Type_Definitions."Idle" ("Enum") w244 w257 State_Type_Definitions."Shutdown" ("Enum") w321 w358 w400 w446 w501 w540 w592 w624] -> w228
              tunnel: w227 -> [_ _ w247 w261 _ w326 w368 w409 w450 w499 w544 w589 w631]
              tunnel: w226 -> [_ _ _ w260 _ w325 w367 w408 w449 w498 w536 w588 w629]
              tunnel: w225 -> [_ _ w246 w256 _ w324 w366 w407 w448 w497 w535 w587 w630]
              tunnel: w214 -> [_ _ _ _ _ w318 w357 w404 w444 w500 w541 w590 w627]
              tunnel: w224 -> [_ _ _ _ _ _ _ _ _ _ _ _ _]
              tunnel: w223 -> [_ _ _ _ _ _ w364 _ w442 w490 w546 _ _]
              tunnel: w222 -> [_ _ _ _ _ _ w363 _ w443 w491 w545 _ _]
              tunnel: w220 -> [_ _ _ _ _ _ _ w406 _ _ _ _ _]
              tunnel: w219 -> [_ _ _ _ _ w317 _ _ _ _ _ _ _]
              tunnel: w218 -> [_ _ _ _ _ _ _ _ _ w486 _ _ _]
              tunnel: w217 -> [_ _ _ _ _ _ _ _ _ _ _ _ _]
              tunnel: [State_Type_Definitions."Idle" ("Enum") State_Type_Definitions."Idle" ("Enum") State_Type_Definitions."Idle" ("Enum") State_Type_Definitions."Idle" ("Enum") State_Type_Definitions."Shutdown" ("Enum") w314 w354 w397 w437 w485 w538 w593 w625] -> w213
              tunnel: w212 -> [_ _ w244 _ _ _ _ _ _ _ _ _ _]
              tunnel: w208 -> [_ _ _ _ _ _ _ _ _ _ _ _ w626]
              tunnel: w211 -> [_ _ _ _ _ _ _ _ _ _ _ _ _]
              tunnel: w210 -> [_ _ _ _ _ _ _ _ _ _ _ _ _]
              tunnel: w207 -> [_ _ _ _ _ _ _ _ _ _ _ _ _]
              tunnel: w206 -> [_ _ _ _ _ _ _ _ _ _ _ w585 _]
              frame 0 {
              }
              frame 1 {
                n107 = for {
                  shift-right: [w243] -> w237
                  shift-left: w240 -> [w242]
                  tunnel: string[] ["INIT", "NAVX CALIBRATE", "RESET FLAGS", "RESET YAW", "RESET ARM"] -> [w241] mode=indexing
                  n108 = Enqueue Element(queue=w242, element=w241) -> (queue out=w243:refnum<queue>)  [unwired: 2 in, 2 out]
                }
              }
              frame 3 {
                n109 = Flush Queue(queue=w247, error in (no error)=w246) -> ()  [unwired: 3 out]
                n110 = for {
                  shift-right: [w253] -> w248
                  shift-left: w249 -> [w252]
                  tunnel: string[] ["STOP", "RESET ENCODERS", "RESET YAW", "ARDUINO MODE 0", "CAM CLOSE", "RESET ARM"] -> [w251] mode=indexing
                  n111 = Enqueue Element(queue=w252, element=w251) -> (queue out=w253:refnum<queue>)  [unwired: 2 in, 2 out]
                }
              }
              frame 4, Default {
                (unwired) TRUE ("Green LED")
                n112 = Dequeue Element(queue=w261, timeout in ms (-1)=w260, error in (no error)=w256) -> (element=w259:T10)  [unwired: 3 out]
                n113 = case shown="\"Start Task 6\"" w259 {
                  tunnel: [w263 w270 w277 w284 w291 w298 w300] -> w255
                  tunnel: w258 -> [w264 w271 w278 w285 w292 w298 w301]
                  tunnel: [State_Type_Definitions."Task 1" ("Enum") State_Type_Definitions."Task 2" ("Enum") State_Type_Definitions."Task 3" ("Enum") State_Type_Definitions."Task 4_A" ("Enum") State_Type_Definitions."Task 6_A" ("Enum") State_Type_Definitions."Idle" ("Enum") State_Type_Definitions."Shutdown" ("Enum")] -> w257
                  frame "Start Task 1" {
                    n114 = for {
                      shift-right: [w268] -> w263
                      shift-left: w264 -> [w267]
                      tunnel: string[] ["RESET ENCODERS", "RESET YAW", "FORWARD", "READ ENCODERS"] -> [w266] mode=indexing
                      n115 = Enqueue Element(queue=w267, element=w266) -> (queue out=w268:refnum<queue>)  [unwired: 2 in, 2 out]
                    }
                  }
                  frame "Start Task 2" {
                    n116 = for {
                      shift-right: [w275] -> w270
                      shift-left: w271 -> [w274]
                      tunnel: string[] ["RESET ENCODERS", "RESET YAW", "ULTRASONIC READ", "ARDUINO MODE 0"] -> [w273] mode=indexing
                      n117 = Enqueue Element(queue=w274, element=w273) -> (queue out=w275:refnum<queue>)  [unwired: 2 in, 2 out]
                    }
                  }
                  frame "Start Task 3" {
                    n118 = for {
                      shift-right: [w282] -> w277
                      shift-left: w278 -> [w281]
                      tunnel: string[] ["RESET ENCODERS", "READ ENCODERS", "R-ACW"] -> [w280] mode=indexing
                      n119 = Enqueue Element(queue=w281, element=w280) -> (queue out=w282:refnum<queue>)  [unwired: 2 in, 2 out]
                    }
                  }
                  frame "Start Task 4" {
                    n120 = for {
                      shift-right: [w289] -> w284
                      shift-left: w285 -> [w288]
                      tunnel: string[] ["STOP", "RESET YAW", "RESET ENCODERS", "ARDUINO MODE 0", "ULTRASONIC READ", "FORWARD"] -> [w287] mode=indexing
                      n121 = Enqueue Element(queue=w288, element=w287) -> (queue out=w289:refnum<queue>)  [unwired: 2 in, 2 out]
                    }
                  }
                  frame "Start Task 6" {
                    n122 = for {
                      shift-right: [w296] -> w291
                      shift-left: w292 -> [w295]
                      tunnel: string[] ["Z STEPPER CAM HEIGHT ", "READ STEPPER VALUES", "OPEN LOG CAM", "", "", ""] -> [w294] mode=indexing
                      n123 = Enqueue Element(queue=w295, element=w294) -> (queue out=w296:refnum<queue>)  [unwired: 2 in, 2 out]
                    }
                  }
                  frame "None", Default {
                  }
                  frame "Exit" {
                    n124 = for {
                      shift-right: [w305] -> w300
                      shift-left: w301 -> [w304]
                      tunnel: string[] ["STOP", "RESET ENCODERS", "RESET YAW", "EXIT"] -> [w303] mode=indexing
                      n125 = Enqueue Element(queue=w304, element=w303) -> (queue out=w305:refnum<queue>)  [unwired: 2 in, 2 out]
                    }
                  }
                }
              }
              frame 5 {
                n126 = for {
                  shift-right: [w313] -> w307
                  shift-left: w309 -> [w312]
                  tunnel: string[] ["INIT", "RESET ENCODERS", "RESET FLAGS", "EXIT"] -> [w311] mode=indexing
                  n127 = Enqueue Element(queue=w312, element=w311) -> (queue out=w313:refnum<queue>)  [unwired: 2 in, 2 out]
                }
              }
              frame 6 {
                # "Use 250"
                n128 = Dequeue Element(queue=w326, timeout in ms (-1)=w325, error in (no error)=w324) -> (element=w323:T10)  [unwired: 3 out]
                n129 = Greater?(x=w317, y=250.0) -> (0:w315:bool)
                n130 = Or(x=w315, y=w318) -> (x .or. y?=w322:bool)
                n131 = case shown="\"None\", Default" w323 {
                  tunnel: w322 -> [w329 _]
                  tunnel: [w333 State_Type_Definitions."True Stop" ("Enum")] -> w321
                  tunnel: w320 -> [w330 w348]
                  tunnel: [w328 w347] -> w319
                  tunnel: [State_Type_Definitions."Idle" ("Enum") State_Type_Definitions."Shutdown" ("Enum")] -> w314
                  frame "None", Default {
                    n132 = case shown="True" w329 {
                      tunnel: w330 -> [w336 w342]
                      tunnel: [w335 w340] -> w328
                      frame False {
                        n133 = for {
                          shift-right: [w338] -> w335
                          shift-left: w336 -> [w339]
                          tunnel: string[] ["READ ENCODERS", "FORWARD"] ("element") -> [w337] mode=indexing
                          n134 = Enqueue Element(queue=w339, element=w337) -> (queue out=w338:refnum<queue>)  [unwired: 2 in, 2 out]
                        }
                      }
                      frame True {
                        n135 = for {
                          shift-right: [w344] -> w340
                          shift-left: w342 -> [w345]
                          tunnel: string[] ["RESET YAW", "RESET ENCODERS", "STOP", "ARDUINO MODE 0"] -> [w343] mode=indexing
                          n136 = Enqueue Element(queue=w345, element=w343) -> (queue out=w344:refnum<queue>)  [unwired: 2 in, 2 out]
                        }
                      }
                    }
                    n137 = Select(t=State_Type_Definitions."True Stop" ("Enum"), s=w329, f=State_Type_Definitions."Task 1" ("Enum")) -> (s? t:f=w333:u16)
                  }
                  frame "Exit" {
                    n138 = for {
                      shift-right: [w352] -> w347
                      shift-left: w348 -> [w353]
                      tunnel: string[] ["STOP", "RESET ENCODERS", "RESET YAW", ""] -> [w351] mode=indexing
                      n139 = Enqueue Element(queue=w353, element=w351) -> (queue out=w352:refnum<queue>)  [unwired: 2 in, 2 out]
                    }
                  }
                }
              }
              frame 7 {
                w362 = u16 10 ("y")
                # ">>Object detected>>"
                n140 = Dequeue Element(queue=w368, timeout in ms (-1)=w367, error in (no error)=w366) -> (element=w365:T10)  [unwired: 3 out]
                n141 = Less?(x=w364, y=w362) -> (x < y?=w361:bool)
                n142 = Less?(x=w363, y=w362) -> (x < y?=w360:bool)
                n143 = Or(x=w361, y=w360) -> (x .or. y?=w359:bool)
                "Object detected?" <- w359
                n144 = case shown="\"None\", Default" w365 {
                  tunnel: w359 -> [w372 _]
                  tunnel: [w374 State_Type_Definitions."True Stop" ("Enum")] -> w358
                  tunnel: w357 -> [w373 _]
                  tunnel: w356 -> [w371 w391]
                  tunnel: [w370 w392] -> w355
                  tunnel: [State_Type_Definitions."Idle" ("Enum") State_Type_Definitions."Shutdown" ("Enum")] -> w354
                  frame "None", Default {
                    n145 = case shown="True" w372 {
                      tunnel: w371 -> [w378 w385]
                      tunnel: [w379 w384] -> w370
                      frame False {
                        n146 = for {
                          tunnel: string[] ["ULTRASONIC READ", "STOP"] ("element") -> [w380] mode=indexing
                          shift-right: [w382] -> w379
                          shift-left: w378 -> [w381]
                          n147 = Enqueue Element(queue=w381, element=w380) -> (queue out=w382:refnum<queue>)  [unwired: 2 in, 2 out]
                        }
                      }
                      frame True {
                        n148 = for {
                          shift-right: [w387] -> w384
                          shift-left: w385 -> [w388]
                          tunnel: string[] ["REVERSE", "ULTRASONIC READ"] -> [w386] mode=indexing
                          n149 = Enqueue Element(queue=w388, element=w386) -> (queue out=w387:refnum<queue>)  [unwired: 2 in, 2 out]
                        }
                      }
                    }
                    n150 = Select(t=State_Type_Definitions."True Stop" ("Enum"), s=w373, f=State_Type_Definitions."Task 2" ("Enum")) -> (s? t:f=w374:u16)
                  }
                  frame "Exit" {
                    n151 = for {
                      shift-right: [w395] -> w392
                      shift-left: w391 -> [w396]
                      tunnel: string[] ["STOP", "RESET ENCODERS", "RESET YAW", "ARDUINO MODE 0"] -> [w394] mode=indexing
                      n152 = Enqueue Element(queue=w396, element=w394) -> (queue out=w395:refnum<queue>)  [unwired: 2 in, 2 out]
                    }
                  }
                }
              }
              frame 10 {
                n153 = Dequeue Element(queue=w409, timeout in ms (-1)=w408, error in (no error)=w407) -> (element=w398:T10)  [unwired: 3 out]
                n154 = Greater?(x=w406, y=150.0) -> (0:w403:bool)
                n155 = Or(x=w403, y=w404) -> (x .or. y?=w399:bool)
                n156 = case shown="\"Exit\"" w398 {
                  tunnel: w399 -> [w412 _]
                  tunnel: [w416 State_Type_Definitions."True Stop" ("Enum")] -> w400
                  tunnel: w402 -> [w413 w432]
                  tunnel: [w411 w431] -> w401
                  tunnel: [State_Type_Definitions."Idle" ("Enum") State_Type_Definitions."Shutdown" ("Enum")] -> w397
                  frame "None", Default {
                    n157 = case shown="False" w412 {
                      tunnel: w413 -> [w419 w425]
                      tunnel: [w418 w423] -> w411
                      frame False {
                        n158 = for {
                          shift-right: [w421] -> w418
                          shift-left: w419 -> [w422]
                          tunnel: string[] ["READ ENCODERS", "R-ACW"] ("element") -> [w420] mode=indexing
                          n159 = Enqueue Element(queue=w422, element=w420) -> (queue out=w421:refnum<queue>)  [unwired: 2 in, 2 out]
                        }
                      }
                      frame True {
                        n160 = for {
                          shift-right: [w427] -> w423
                          shift-left: w425 -> [w428]
                          tunnel: string[] ["RESET YAW", "RESET ENCODERS", "STOP", "ARDUINO MODE 0"] -> [w426] mode=indexing
                          n161 = Enqueue Element(queue=w428, element=w426) -> (queue out=w427:refnum<queue>)  [unwired: 2 in, 2 out]
                        }
                      }
                    }
                    n162 = Select(t=State_Type_Definitions."True Stop" ("Enum"), s=w412, f=State_Type_Definitions."Task 3" ("Enum")) -> (s? t:f=w416:T9)
                  }
                  frame "Exit" {
                    n163 = for {
                      shift-right: [w435] -> w431
                      shift-left: w432 -> [w436]
                      tunnel: string[] ["STOP", "RESET ENCODERS", "RESET YAW", ""] -> [w434] mode=indexing
                      n164 = Enqueue Element(queue=w436, element=w434) -> (queue out=w435:refnum<queue>)  [unwired: 2 in, 2 out]
                    }
                  }
                }
              }
              frame 11 {
                w441 = 20
                # ">> Outputs true if object detected >>"
                # ">> Manual override >>"
                n165 = Dequeue Element(queue=w450, timeout in ms (-1)=w449, error in (no error)=w448) -> (element=w447:T10)  [unwired: 3 out]
                n166 = Less?(x=w443, y=w441) -> (x < y?=w439:bool)
                n167 = Less?(x=w442, y=w441) -> (x < y?=w440:bool)
                n168 = And(x=w440, y=w439) -> (x .and. y?=w438:bool)
                "Detect?" <- w438
                n169 = case shown="\"None\", Default" w447 {
                  tunnel: [w460 State_Type_Definitions."True Stop" ("Enum")] -> w446
                  tunnel: [w458 w479] -> w445
                  tunnel: w451 -> [w457 _]
                  tunnel: w444 -> [w455 _]
                  tunnel: w438 -> [w453 _]
                  tunnel: [w452 State_Type_Definitions."Shutdown" ("Enum")] -> w437
                  frame "None", Default {
                    # ">> WIill proceed to part ii if not manual override >>"
                    # ">>If ENABLE or Trigger is set to true>>"
                    n170 = Or(x=w453, y=w455) -> (x .or. y?=w454:bool)
                    n171 = case shown="False" w454 {
                      tunnel: [w467 w472] -> w458
                      tunnel: w457 -> [w465 w471]
                      frame False {
                        n172 = for {
                          shift-right: [w469] -> w467
                          shift-left: w465 -> [w470]
                          tunnel: string[] ["FORWARD", "ULTRASONIC READ", ""] ("element") -> [w468] mode=indexing
                          n173 = Enqueue Element(queue=w470, element=w468) -> (queue out=w469:refnum<queue>)  [unwired: 2 in, 2 out]
                        }
                      }
                      frame True {
                        n174 = for {
                          shift-right: [w475] -> w472
                          shift-left: w471 -> [w476]
                          tunnel: string[] ["STOP", "RESET ENCODERS", "RESET YAW", "ARDUINO MODE 0"] -> [w474] mode=indexing
                          n175 = Enqueue Element(queue=w476, element=w474) -> (queue out=w475:refnum<queue>)  [unwired: 2 in, 2 out]
                        }
                      }
                    }
                    n176 = case shown="False" w455 {
                      tunnel: [State_Type_Definitions."True Stop" ("Enum") State_Type_Definitions."True Stop" ("Enum")] -> w456
                      tunnel: [State_Type_Definitions."Task 4_B" ("Enum") State_Type_Definitions."Idle" ("Enum")] -> w452
                      frame False {
                      }
                      frame True {
                      }
                    }
                    n177 = Select(t=w456, s=w454, f=State_Type_Definitions."Task 4_A" ("Enum")) -> (s? t:f=w460:T9)
                  }
                  frame "Exit" {
                    n178 = for {
                      shift-right: [w482] -> w479
                      shift-left: _ -> [w483]
                      tunnel: string[] ["STOP", "RESET ENCODERS", "RESET YAW", ""] -> [w481] mode=indexing
                      n179 = Enqueue Element(queue=w483, element=w481) -> (queue out=w482:refnum<queue>)  [unwired: 2 in, 2 out]
                    }
                  }
                }
              }
              frame 12 {
                w494 = 20
                # ">> Outputs true if 150 mm has been moved >>"
                # ">> Outputs true if sensor not obstructed>>"
                # ">> Manual override >>"
                n180 = Dequeue Element(queue=w499, timeout in ms (-1)=w498, error in (no error)=w497) -> (element=w496:T10)  [unwired: 3 out]
                n181 = Greater?(x=w491, y=w494) -> (0:w492:bool)
                n182 = Greater?(x=w490, y=w494) -> (0:w493:bool)
                n183 = Greater Or Equal?(x=w486, y=80.0) -> (x >= y?=w488:bool)
                n184 = And(x=w493, y=w492) -> (x .and. y?=w487:bool)
                n185 = And(x=w488, y=w487) -> (x .and. y?=w484:bool)
                n186 = case shown="\"None\", Default" w496 {
                  tunnel: [w511 State_Type_Definitions."True Stop" ("Enum")] -> w501
                  tunnel: [w509 w530] -> w502
                  tunnel: w495 -> [w508 _]
                  tunnel: w500 -> [w506 _]
                  tunnel: w484 -> [w504 _]
                  tunnel: [w503 State_Type_Definitions."Shutdown" ("Enum")] -> w485
                  frame "None", Default {
                    # ">> WIill proceed to part ii if not manual override >>"
                    # ">>If ENABLE or Trigger is set to true>>"
                    n187 = Or(x=w504, y=w506) -> (x .or. y?=w505:bool)
                    n188 = case shown="False" w505 {
                      tunnel: [w518 w523] -> w509
                      tunnel: w508 -> [w516 w522]
                      frame False {
                        n189 = for {
                          shift-right: [w520] -> w518
                          shift-left: w516 -> [w521]
                          tunnel: string[] ["RIGHT", "ULTRASONIC READ", "READ ENCODERS"] ("element") -> [w519] mode=indexing
                          n190 = Enqueue Element(queue=w521, element=w519) -> (queue out=w520:refnum<queue>)  [unwired: 2 in, 2 out]
                        }
                      }
                      frame True {
                        n191 = for {
                          shift-right: [w526] -> w523
                          shift-left: w522 -> [w527]
                          tunnel: string[] ["STOP", "RESET ENCODERS", "RESET YAW", "ARDUINO MODE 0"] -> [w525] mode=indexing
                          n192 = Enqueue Element(queue=w527, element=w525) -> (queue out=w526:refnum<queue>)  [unwired: 2 in, 2 out]
                        }
                      }
                    }
                    n193 = case shown="True" w506 {
                      tunnel: [State_Type_Definitions."True Stop" ("Enum") State_Type_Definitions."True Stop" ("Enum")] -> w507
                      tunnel: [State_Type_Definitions."Task 4_C" ("Enum") State_Type_Definitions."Idle" ("Enum")] -> w503
                      frame False {
                      }
                      frame True {
                      }
                    }
                    n194 = Select(t=w507, s=w505, f=State_Type_Definitions."Task 4_B" ("Enum")) -> (s? t:f=w511:T9)
                  }
                  frame "Exit" {
                    n195 = for {
                      shift-right: [w533] -> w530
                      shift-left: _ -> [w534]
                      tunnel: string[] ["STOP", "RESET ENCODERS", "RESET YAW", ""] -> [w532] mode=indexing
                      n196 = Enqueue Element(queue=w534, element=w532) -> (queue out=w533:refnum<queue>)  [unwired: 2 in, 2 out]
                    }
                  }
                }
              }
              frame 13 {
                w549 = 20
                # ">> Outputs true if object detected >>"
                # ">> Manual override >>"
                n197 = Dequeue Element(queue=w544, timeout in ms (-1)=w536, error in (no error)=w535) -> (element=w537:T10)  [unwired: 3 out]
                n198 = Less?(x=w545, y=w549) -> (x < y?=w547:bool)
                n199 = Less?(x=w546, y=w549) -> (x < y?=w548:bool)
                n200 = And(x=w548, y=w547) -> (x .and. y?=w542:bool)
                n201 = case shown="\"None\", Default" w537 {
                  tunnel: [w558 State_Type_Definitions."True Stop" ("Enum")] -> w540
                  tunnel: [w556 w578] -> w539
                  tunnel: w543 -> [w555 w575]
                  tunnel: w541 -> [w553 _]
                  tunnel: w542 -> [w551 _]
                  tunnel: [w550 State_Type_Definitions."Shutdown" ("Enum")] -> w538
                  frame "None", Default {
                    # ">> WIill proceed to part ii if not manual override >>"
                    # ">>If ENABLE or Trigger is set to true>>"
                    n202 = Or(x=w551, y=w553) -> (x .or. y?=w552:bool)
                    n203 = case shown="False" w552 {
                      tunnel: [w565 w570] -> w556
                      tunnel: w555 -> [w563 w569]
                      frame False {
                        n204 = for {
                          shift-right: [w567] -> w565
                          shift-left: w563 -> [w568]
                          tunnel: string[] ["FORWARD", "ULTRASONIC READ", ""] ("element") -> [w566] mode=indexing
                          n205 = Enqueue Element(queue=w568, element=w566) -> (queue out=w567:refnum<queue>)  [unwired: 2 in, 2 out]
                        }
                      }
                      frame True {
                        n206 = for {
                          shift-right: [w573] -> w570
                          shift-left: w569 -> [w574]
                          tunnel: string[] ["STOP", "RESET ENCODERS", "RESET YAW", "ARDUINO MODE 0"] -> [w572] mode=indexing
                          n207 = Enqueue Element(queue=w574, element=w572) -> (queue out=w573:refnum<queue>)  [unwired: 2 in, 2 out]
                        }
                      }
                    }
                    n208 = case shown="True" w553 {
                      tunnel: [State_Type_Definitions."True Stop" ("Enum") State_Type_Definitions."True Stop" ("Enum")] -> w554
                      tunnel: [State_Type_Definitions."Idle" ("Enum") State_Type_Definitions."Idle" ("Enum")] -> w550
                      frame False {
                      }
                      frame True {
                      }
                    }
                    n209 = Select(t=w554, s=w552, f=State_Type_Definitions."Task 4_C" ("Enum")) -> (s? t:f=w558:T9)
                  }
                  frame "Exit" {
                    n210 = for {
                      shift-right: [w581] -> w578
                      shift-left: w575 -> [w582]
                      tunnel: string[] ["STOP", "RESET ENCODERS", "RESET YAW", ""] -> [w580] mode=indexing
                      n211 = Enqueue Element(queue=w582, element=w580) -> (queue out=w581:refnum<queue>)  [unwired: 2 in, 2 out]
                    }
                  }
                }
              }
              frame 23 {
                (unwired) u16 10 ("y")
                n212 = Dequeue Element(queue=w589, timeout in ms (-1)=w588, error in (no error)=w587) -> (element=w594:T10)  [unwired: 3 out]
                n213 = Equal?(x=w585, y=u8 100) -> (x = y?=w584:bool)
                n214 = case shown="\"None\", Default" w594 {
                  tunnel: [w601 State_Type_Definitions."True Stop" ("Enum")] -> w592
                  tunnel: [w600 w618] -> w591
                  tunnel: [State_Type_Definitions."Idle" ("Enum") State_Type_Definitions."Shutdown" ("Enum")] -> w593
                  tunnel: w590 -> [w596 _]
                  tunnel: w586 -> [w598 _]
                  tunnel: w584 -> [w595 _]
                  frame "None", Default {
                    n215 = case shown="False" w595 {
                      tunnel: [w606 w612] -> w600
                      tunnel: w598 -> [w604 w610]
                      frame False {
                        n216 = for {
                          tunnel: string[] ["Z STEPPER CAM HEIGHT", "READ STEPPER VALUES"] ("element") -> [w607] mode=indexing
                          shift-right: [w609] -> w606
                          shift-left: w604 -> [w608]
                          n217 = Enqueue Element(queue=w608, element=w607) -> (queue out=w609:refnum<queue>)  [unwired: 2 in, 2 out]
                        }
                      }
                      frame True {
                        n218 = for {
                          shift-right: [w614] -> w612
                          shift-left: w610 -> [w615]
                          tunnel: string[] ["CAM ACQ", ""] -> [w613] mode=indexing
                          n219 = Enqueue Element(queue=w615, element=w613) -> (queue out=w614:refnum<queue>)  [unwired: 2 in, 2 out]
                        }
                      }
                    }
                    n220 = Or(x=w595, y=w596) -> (x .or. y?=w597:bool)
                    n221 = Select(t=State_Type_Definitions."Task 6_B" ("Enum"), s=w597, f=State_Type_Definitions."Task 6_A" ("Enum")) -> (s? t:f=w601:T9)
                  }
                  frame "Exit" {
                    n222 = for {
                      shift-right: [w621] -> w618
                      shift-left: _ -> [w622]
                      tunnel: string[] ["STOP", "RESET ENCODERS", "RESET YAW", "ARDUINO MODE 0"] -> [w620] mode=indexing
                      n223 = Enqueue Element(queue=w622, element=w620) -> (queue out=w621:refnum<queue>)  [unwired: 2 in, 2 out]
                    }
                  }
                }
              }
              frame 24 {
                n224 = Dequeue Element(queue=w631, timeout in ms (-1)=w629, error in (no error)=w630) -> (element=w628:T10)  [unwired: 3 out]
                n225 = case shown="\"None\", Default" w628 {
                  tunnel: [w638 State_Type_Definitions."True Stop" ("Enum")] -> w624
                  tunnel: [w637 w655] -> w632
                  tunnel: [State_Type_Definitions."Idle" ("Enum") State_Type_Definitions."Shutdown" ("Enum")] -> w625
                  tunnel: w627 -> [w633 _]
                  tunnel: w626 -> [w635 _]
                  tunnel: w623 -> [w634 _]
                  frame "None", Default {
                    n226 = case shown="True" w635 {
                      tunnel: [w643 w649] -> w637
                      tunnel: w634 -> [w642 w647]
                      frame False {
                        n227 = for {
                          shift-right: [w646] -> w643
                          shift-left: w642 -> [w645]
                          tunnel: string[] ["CAM ACQ", "OPEN CLAW"] -> [w644] mode=indexing
                          n228 = Enqueue Element(queue=w645, element=w644) -> (queue out=w646:refnum<queue>)  [unwired: 2 in, 2 out]
                        }
                      }
                      frame True {
                        n229 = for {
                          shift-right: [w651] -> w649
                          shift-left: w647 -> [w652]
                          tunnel: string[] ["CAM ACQ", "CLOSE CLAW"] -> [w650] mode=indexing
                          n230 = Enqueue Element(queue=w652, element=w650) -> (queue out=w651:refnum<queue>)  [unwired: 2 in, 2 out]
                        }
                      }
                    }
                    n231 = Select(t=State_Type_Definitions."True Stop" ("Enum"), s=w633, f=State_Type_Definitions."Task 6_B" ("Enum")) -> (s? t:f=w638:T9)
                  }
                  frame "Exit" {
                    n232 = for {
                      shift-right: [w658] -> w655
                      shift-left: _ -> [w659]
                      tunnel: string[] ["STOP", "RESET ENCODERS", "RESET YAW", "ARDUINO MODE 0"] -> [w657] mode=indexing
                      n233 = Enqueue Element(queue=w659, element=w657) -> (queue out=w658:refnum<queue>)  [unwired: 2 in, 2 out]
                    }
                  }
                }
              }
            }
          }
        }
      }
      n234 = call <vilib>:"DIO Close.vi"("error in (no error)"=w22, "DIO Info In"=w25) -> ()  [unwired: 9 in, 1 out]
      n235 = call <vilib>:"DIO Close.vi"("error in (no error)"=w32, "DIO Info In"=w34) -> ()  [unwired: 9 in, 1 out]
      n236 = call <vilib>:"NavX Close.vi"("error in (no error)"=w20, "NavX Info In"=w21) -> ()  [unwired: 9 in, 1 out]
      n237 = call <vilib>:"DIO Close.vi"("error in (no error)"=w27, "DIO Info In"=w29) -> ()  [unwired: 9 in, 1 out]
      n238 = call <vilib>:"DIO Close.vi"("error in (no error)"=w8, "DIO Info In"=w9) -> ()  [unwired: 9 in, 1 out]
      n239 = call <vilib>:"DIO Close.vi"("error in (no error)"=w3, "DIO Info In"=w4) -> ()  [unwired: 9 in, 1 out]
      n240 = while {
        stop <- w70 stop-if-true
        n241 = call <vilib>:"RT Get CPU Loads.vi"() -> ("CPU loads"=→"CPU loads":T2[])  [unwired: 10 in, 1 out]
        n242 = Wait (ms)(milliseconds to wait=u32 100) -> ()  [unwired: 1 out]
        n243 = call "FGV Bool.vi"("Init/Read/Write State"=States_for_Action_Engine."Read") -> ("Output node"=w70:bool)  [unwired: 2 in, 1 out]
      }
      n244 = Merge Errors "Merge Errors"(w62, w61) -> (w44:errorcluster)
      n245 = Merge Errors(w48, w44) -> (w43:errorcluster)
      n246 = Destroy User Event(user event=w65, error in=w43) -> ()  [unwired: 1 out]
      n247 = Destroy User Event(user event=w66, error in=w43) -> ()  [unwired: 1 out]
      n248 = Unregister For Events(event registration refnum=w57, error in=w43) -> ()  [unwired: 1 out]
      n249 = Release Queue(queue=w39, error in (no error)=w43) -> (error out=w19:errorcluster)  [unwired: 1 in, 2 out]
      n250 = Release Queue(queue=w56, error in (no error)=w43) -> ()  [unwired: 1 in, 3 out]
      n251 = call <vilib>:"Simple Error Handler.vi"("error in (no error)"=w19) -> ("error out"=w18:errorcluster)  [unwired: 4 in, 4 out]
      n252 = call <vilib>:"Reset myRIO.vi"("error in (no error)"=w18) -> ("error out"=→"error out":errorcluster)  [unwired: 10 in]
    }
    frame #2 {
      n253 = call "Imaq Dispose"("All Images? (No)"=TRUE) -> ()  [unwired: 5 in, 1 out]
      n254 = Wait (ms)(milliseconds to wait=u32 100) -> ()  [unwired: 1 out]
    }
  }
